vi "Vision_Right_R3.3.vi"() -> ()   [LabVIEW 2015]
uses:
  <vilib>/vision/Pattern Matching.llb/IMAQ Curve Parameters.ctl
  <vilib>/vision/Pattern Matching.llb/IMAQ Match Range Setting.ctl
  <vilib>/userdefined/High Color/IMAQdx.ctl
  <vilib>/vision/driver/NI_Vision_Acquisition_Software.lvlib
  <vilib>/vision/NI_Vision_Development_Module.lvlib
panel:
  in  "Range 0 Default\nSetting Values":T1={"Min Scale"=50.0, "Max Scale"=160.0, "Min Score"=850.0, "Lower Transition Scale"=45.0, "Upper Transition Scale"=200.0, "ROI Vertical"=2.0, "ROI Horizontal"=1.0, "Scale Cushion"=15.0, "Curve Parameters"={"Min Length"=15, "Row Search Step"=10, "Col Search Step"=10}, "Beacon Cushion (px)"=3.0, "Max Scale Diff\nfrom Main"=50.0}
  in  "Range 0 Templates":T2={"Sub - 2 File Path"=path "/home/lvuser/Beacon_Templates/Range_0/Range 0.png", "Sub Beacon Template File Path - ARRAY"=[path "/home/lvuser/Beacon_Templates/Range_1/Sub 0 - Range 1.png", path "/home/lvuser/Beacon_Templates/Range_1/Sub 1 - Range 1.png", path "/home/lvuser/Beacon_Templates/Range_1/Sub 2 - Range 1.png", path "/home/lvuser/Beacon_Templates/Range_1/Sub 3 - Range 1.png", path "/home/lvuser/Beacon_Templates/Range_1/Sub 4 - Range 1.png"]}
  in  "Correlation Score Threhsold (Range 0)":sgl=750.0
  in  "stop":bool
  in  "select (true= use advanced features\nfase= dont use)":bool
  in  "Range 3 Default\nSetting Values":T1={"Min Scale"=50.0, "Max Scale"=150.0, "Min Score"=800.0, "Lower Transition Scale"=1.0, "Upper Transition Scale"=130.0, "ROI Vertical"=3.5, "ROI Horizontal"=4.0, "Scale Cushion"=15.0, "Curve Parameters"={"Min Length"=2, "Row Search Step"=5, "Col Search Step"=5}, "Beacon Cushion (px)"=5.0, "Max Scale Diff\nfrom Main"=10.0}
  in  "Range 2 Default\nSetting Values":T1={"Min Scale"=65.0, "Max Scale"=130.0, "Min Score"=800.0, "Lower Transition Scale"=65.0, "Upper Transition Scale"=125.0, "ROI Vertical"=2.8, "ROI Horizontal"=4.0, "Scale Cushion"=17.0, "Curve Parameters"={"Min Length"=10, "Row Search Step"=10, "Col Search Step"=10}, "Beacon Cushion (px)"=15.0, "Max Scale Diff\nfrom Main"=20.0}
  in  "No Lock Default\nSetting Values":T3={"Min Scale"=25.0, "Max Scale"=200.0, "Min Score"=750.0, "Lower Transition Scale"=35.0, "Upper Transition Scale"=250.0, "ROI Vertical"=15.0, "ROI Horizontal"=15.0, "Scale Cushion"=15.0, "Curve Parameters"={"Min Length"=5, "Row Search Step"=10, "Col Search Step"=10}, "Scale Cushion 2"=15.0, "Max Scale Diff\nfrom Main"=15.0}
  in  "ROI Decay Factor (px)":dbl=50.0
  in  "ROBOT STATE\n(fwd, bwd, neither) 2":i32
  in  "Score Decay \nFactor 2":dbl=50.0
  in  "Range 1 Default\nSetting Values":T1={"Min Scale"=25.0, "Max Scale"=100.0, "Min Score"=800.0, "Lower Transition Scale"=35.0, "Upper Transition Scale"=67.0, "ROI Vertical"=0.75, "ROI Horizontal"=5.0, "Scale Cushion"=23.0, "Curve Parameters"={"Min Length"=15, "Row Search Step"=15, "Col Search Step"=15}, "Beacon Cushion (px)"=25.0, "Max Scale Diff\nfrom Main"=25.0}
  out "Next Template":T4(ring)
  out "Current Template":T4(ring)
  in  "Initial Template":T4(ring)
  in  "Range 3 Templates":T2={"Sub - 2 File Path"=path "/home/lvuser/Beacon_Templates/Range_3/5 Beacons - Range 3.png", "Sub Beacon Template File Path - ARRAY"=[path "/home/lvuser/Beacon_Templates/Range_3/Sub 0 - Range 3.png", path "/home/lvuser/Beacon_Templates/Range_3/Sub 1 - Range 3.png", path "/home/lvuser/Beacon_Templates/Range_3/Sub 2 - Range 3.png", path "/home/lvuser/Beacon_Templates/Range_3/Sub 3 - Range 3.png", path "/home/lvuser/Beacon_Templates/Range_3/Sub 4 - Range 3.png"]}
  in  "Range 2 Templates":T2={"Sub - 2 File Path"=path "/home/lvuser/Beacon_Templates/Range_2/5 Beacons - Range 2.png", "Sub Beacon Template File Path - ARRAY"=[path "/home/lvuser/Beacon_Templates/Range_2/Sub 0 - Range 2.png", path "/home/lvuser/Beacon_Templates/Range_2/Sub 1 - Range 2.png", path "/home/lvuser/Beacon_Templates/Range_2/Sub 2 - Range 2.png", path "/home/lvuser/Beacon_Templates/Range_2/Sub 3 - Range 2.png", path "/home/lvuser/Beacon_Templates/Range_2/Sub 4 - Range 2.png"]}
  in  "Range 1 Templates - RIGHT":T2={"Sub - 2 File Path"=path "/home/lvuser/Beacon_Templates/Range_1/2_Beacons_Right - Range 1.png", "Sub Beacon Template File Path - ARRAY"=[path "/home/lvuser/Beacon_Templates/Range_1/Sub 0 - Range 1.png", path "/home/lvuser/Beacon_Templates/Range_1/Sub 1 - Range 1.png", path "/home/lvuser/Beacon_Templates/Range_1/Sub 2 - Range 1.png", path "/home/lvuser/Beacon_Templates/Range_1/Sub 3 - Range 1.png", path "/home/lvuser/Beacon_Templates/Range_1/Sub 4 - Range 1.png"]}
  out "Current Correlation Score":sgl
  in  "Correlation Score Threhsold":sgl=300.0
  out "New Min Score":dbl=800.0
  out "New Low Scale":dbl=25.0
  out "New high Scale":dbl=100.0
  in  "Absolute\nMinimum Score":dbl=750.0
  in  "Absolute\nMaximum Scale":dbl=250.0
  in  "Absolute\nMinimum Scale":dbl=25.0
  in  "Score\nCushion":dbl=192.0
  in  "Avg Scale - Last":dbl=50.0
  in  "Avg Score - Last":dbl=986.6820373535156
  in  "Max Window\n for Avg":u8=3
  in  "Valid Treshold\nfor Lock":i16=3
  out "Current  Score":sgl
  out "Current  Scale":sgl
  out "Current Valid?":bool
  out "Beacon - Scales":sgl[](array[numeric])
  out "beacon - Scores":sgl[](array[numeric])
  out "Beacons Found":bool[](array[boolean])
  out "Horiztonall Beacon \nCushion (pixels)":sgl=25.0
  out "Tracking Info":T5={"Lock"=FALSE, "Current Valid"=FALSE, "Current Template"=enum."Range 1", "Tracking Coordinates"={"X"=159.0, "Y"=119.0}, "Setting Values"={"Min Score"=800.0, "Min Scale"=25.0, "Max Scale"=100.0, "Curve Parameters"={"Min Length"=15, "Row Search Step"=15, "Col Search Step"=15}}}
  out "dT":u32=629
  out "Avg Scale":dbl=50.0
  out "Avg Score":dbl=986.6820373535156
  out "Current Search Settings":T8={"Curve Parameters"={"Extraction Mode"=1, "Edge Threshold"=200, "Edge Filter Size"=0, "Min Length"=15, "Row Search Step Size"=15, "Col Search Step Size"=15, "Max Endpoint Gap"=4, "Closed"=TRUE, "Subpixel"=TRUE}, "Match Mode"={"Rotation"=TRUE, "Scale"=TRUE, "Occlusion"=TRUE, "Reserved"=FALSE, "Reserved"=FALSE, "Reserved"=FALSE}, "Range Settings"=[{"Match Constraints"=0, "Min"=-10.0, "Max"=2.0}, {"Match Constraints"=1, "Min"=25.0, "Max"=100.0}, {"Match Constraints"=2, "Min"=0.0, "Max"=20.0}], "Number of Matches"=1, "Minimum Match Score"=800.0, "SubPixel Accuracy"=TRUE, "Adv. Geometric Match Options 2"=[{"Setup Data Item"=20, "Item Value"=0.0}, {"Setup Data Item"=22, "Item Value"=1.0}]} {"Curve Parameters"."Extraction Mode" items=["Normal", "Uniform Regions"]; "Curve Parameters"."Edge Filter Size" items=["Fine", "Normal", "Contour Tracing"]; "Curve Parameters"."Max Endpoint Gap" min=0; "Curve Parameters"."Col Search Step Size" min=1 max=255 step=1; "Curve Parameters"."Row Search Step Size" min=1 max=255 step=1; "Curve Parameters"."Min Length" min=0; "Curve Parameters"."Edge Threshold" min=1 max=350 step=1; "Range Settings"."Max" format="%.2f"; "Range Settings"."Min" format="%.2f"; "Range Settings"."Match Constraints" items=["Rotation Angle (degrees)", "Scale Factor (%)", "Occlusion (%)"]}
  out "Valid Scale History":dbl[](array[numeric]) format="%#_13g"
  out "Valid Score History":dbl[](array[numeric]) format="%#_13g"
  out "Valid Beacon History - in":bool[](array[boolean])
  out "Startup Flag":bool
  out "Lock Status":bool
  out "Y Coordinates":sgl[](array[numeric])
  out "X Coordinates":sgl[](array[numeric])
  out "Right Image out":T9(plugin-control)
  in  "History Size":i32=19
  in  "INITIAL Search Settings":T8={"Curve Parameters"={"Extraction Mode"=1, "Edge Threshold"=200, "Edge Filter Size"=0, "Min Length"=15, "Row Search Step Size"=10, "Col Search Step Size"=10, "Max Endpoint Gap"=4, "Closed"=TRUE, "Subpixel"=TRUE}, "Match Mode"={"Rotation"=TRUE, "Scale"=TRUE, "Occlusion"=TRUE, "Reserved"=FALSE, "Reserved"=FALSE, "Reserved"=FALSE}, "Range Settings"=[{"Match Constraints"=0, "Min"=-10.0, "Max"=2.0}, {"Match Constraints"=1, "Min"=25.0, "Max"=150.0}, {"Match Constraints"=2, "Min"=0.0, "Max"=20.0}], "Number of Matches"=1, "Minimum Match Score"=750.0, "SubPixel Accuracy"=TRUE, "Adv. Geometric Match Options 2"=[{"Setup Data Item"=20, "Item Value"=0.0}, {"Setup Data Item"=22, "Item Value"=1.0}]} {"Curve Parameters"."Extraction Mode" items=["Normal", "Uniform Regions"]; "Curve Parameters"."Edge Filter Size" items=["Fine", "Normal", "Contour Tracing"]; "Curve Parameters"."Max Endpoint Gap" min=0; "Curve Parameters"."Col Search Step Size" min=1 max=255 step=1; "Curve Parameters"."Row Search Step Size" min=1 max=255 step=1; "Curve Parameters"."Min Length" min=0; "Curve Parameters"."Edge Threshold" min=1 max=350 step=1; "Range Settings"."Max" format="%.2f"; "Range Settings"."Min" format="%.2f"; "Range Settings"."Match Constraints" items=["Rotation Angle (degrees)", "Scale Factor (%)", "Occlusion (%)"]; "Adv. Geometric Match Options 2"."Setup Data Item" items=["Curve Extraction Mode", "Curve Edge Threshold", "Curve Edge Filter Size", "Min Curve Length", "Curve Row Search Step Size", "Curve Col Search Step Size", "Curve Max Endpoint Gap", "Extract Closed Curves", "Enable Subpixel Curve Extraction", "Enable Correlation Score", "Enable Subpixel Accuracy", "Subpixel Iterations", "Subpixel Tolerance", "Initial Match List Length", "Enable Target Template Curve Score", "Min Match Separation Distance", "Min Match Separation Angle", "Min Match Separation Scale", "Max Match Overlap", "Enable Coarse Result", "Enable Calibration Support", "Enable Contrast Reversal", "Search Strategy", "Refinement Match Factor", "Subpixel Match Factor"]}
  # "ROI Factore (per Template)"
  # "Template Transition Scales"
  # "Search Parameter Limits"
  # "TEMPLATE FILE PATHS"
  # "Config"
  # "Initial Settings"
  # "Range"
  # "Range"
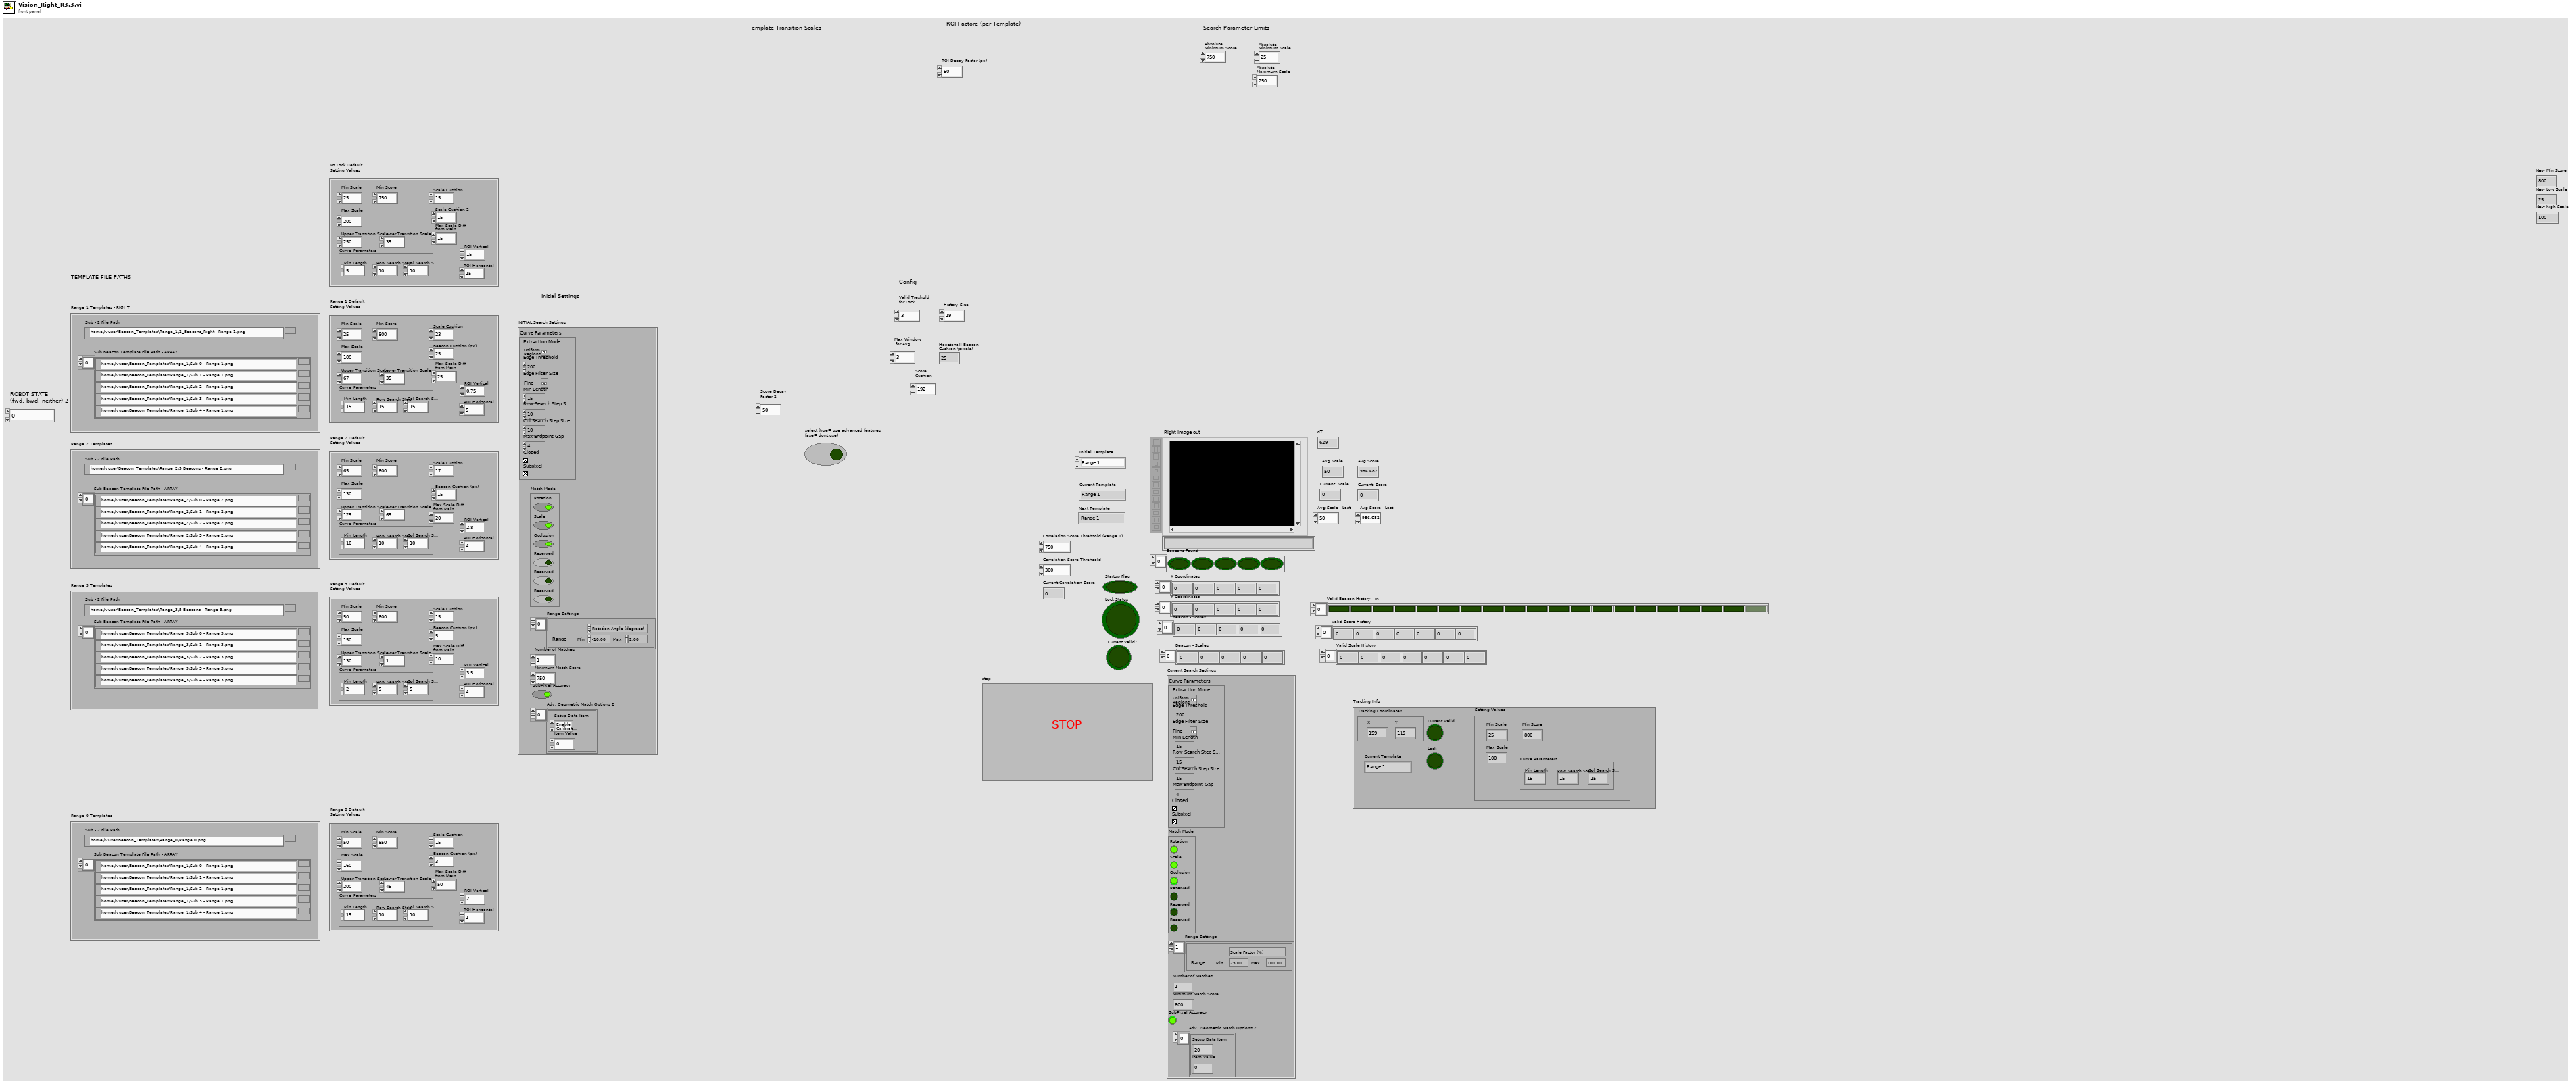
[diagram p1: front panel]
types:
  T1 = cluster{"Min Scale":dbl, "Max Scale":dbl, "Min Score":dbl, "Lower Transition Scale":sgl, "Upper Transition Scale":sgl, "ROI Vertical":dbl, "ROI Horizontal":dbl, "Scale Cushion":dbl, "Curve Parameters":cluster{"Min Length":i32, "Row Search Step":i32, "Col Search Step":i32}, "Beacon Cushion (px)":dbl, "Max Scale Diff\nfrom Main":dbl}
  T2 = cluster{"Sub - 2 File Path":path, "Sub Beacon Template File Path - ARRAY":path[]}
  T3 = cluster{"Min Scale":dbl, "Max Scale":dbl, "Min Score":dbl, "Lower Transition Scale":sgl, "Upper Transition Scale":sgl, "ROI Vertical":dbl, "ROI Horizontal":dbl, "Scale Cushion":dbl, "Curve Parameters":cluster{"Min Length":i32, "Row Search Step":i32, "Col Search Step":i32}, "Scale Cushion 2":dbl, "Max Scale Diff\nfrom Main":dbl}
  T4 = enum16{"Range 1", "Range 2", "Range 3", "Range 0"}
  T5 = cluster{"Lock":bool, "Current Valid":bool, "Current Template":enum16{"Range 1", "Range 2", "Range 3", "Range 0"}, "Tracking Coordinates":cluster{"X":dbl, "Y":dbl}, "Setting Values":cluster{"Min Score":dbl, "Min Scale":dbl, "Max Scale":dbl, "Curve Parameters":cluster{"Min Length":i32, "Row Search Step":i32, "Col Search Step":i32}}}
  T6 = typedef "IMAQ Curve Parameters.ctl" = cluster{"Extraction Mode":u32, "Edge Threshold":i32, "Edge Filter Size":u32, "Min Length":i32, "Row Search Step Size":i32, "Col Search Step Size":i32, "Max Endpoint Gap":i32, "Closed":bool, "Subpixel":bool}
  T7 = typedef "IMAQ Match Range Setting.ctl" = cluster{"Match Constraints":u32, "Min":dbl, "Max":dbl}
  T8 = cluster{"Curve Parameters":T6, "Match Mode":cluster{"Rotation":bool, "Scale":bool, "Occlusion":bool, "Reserved":bool, "Reserved":bool, "Reserved":bool}, "Range Settings":T7[], "Number of Matches":i32, "Minimum Match Score":sgl, "SubPixel Accuracy":bool, "Adv. Geometric Match Options 2":cluster{"Setup Data Item":u16, "Item Value":dbl}[]}
  T9 = typedef "IMAQ Image.ctl" = refnum<image>
  T10 = typedef "IMAQdx.ctl" = refnum<k21>
  T11 = typedef "Image Type" = u32
  T12 = typedef "ROI Descriptor" = cluster{"Global Rectangle":i32[], "Contours":cluster{"ID":enum32{"External", "Internal"}, "Type":u32, "Coordinates":i32[]}[]}
  T13 = typedef "IMAQ GM Match Report.ctl" = cluster{"Position":cluster{"x":sgl, "y":sgl}, "Angle":sgl, "Scale":sgl, "Score":sgl, "Bounding Box":cluster{"x":sgl, "y":sgl}[], "Contrast Reversed":bool, "Occlusion %":sgl, "Template Target Curve Score":sgl, "Target Template Curve Score":sgl, "Correlation Score":sgl}
  T14 = cluster{"Matches[0]":T13, "Matches[1]":T13, "Matches[2]":T13, "Matches[3]":T13, "Matches[4]":T13, "Matches[5]":T13, "Matches[6]":T13, "Matches[7]":T13, "Matches[8]":T13}
  T15 = cluster{"Bounding Box[0]":cluster{"x":sgl, "y":sgl}, "Bounding Box[1]":cluster{"x":sgl, "y":sgl}, "Bounding Box[2]":cluster{"x":sgl, "y":sgl}, "Bounding Box[3]":cluster{"x":sgl, "y":sgl}, "Bounding Box[4]":cluster{"x":sgl, "y":sgl}, "Bounding Box[5]":cluster{"x":sgl, "y":sgl}, "Bounding Box[6]":cluster{"x":sgl, "y":sgl}, "Bounding Box[7]":cluster{"x":sgl, "y":sgl}, "Bounding Box[8]":cluster{"x":sgl, "y":sgl}}
  T16 = cluster{"Matches (Geometric Matching 1)[0]":T13, "Matches (Geometric Matching 1)[1]":T13, "Matches (Geometric Matching 1)[2]":T13, "Matches (Geometric Matching 1)[3]":T13, "Matches (Geometric Matching 1)[4]":T13, "Matches (Geometric Matching 1)[5]":T13, "Matches (Geometric Matching 1)[6]":T13, "Matches (Geometric Matching 1)[7]":T13, "Matches (Geometric Matching 1)[8]":T13}
  T17 = cluster{"Min Length":i32, "Row Search Step":i32, "Col Search Step":i32}
  T18 = cluster{"Extraction Mode":u32, "Edge Threshold":i32, "Edge Filter Size":u32, "Min Length":i32, "Row Search Step":i32, "Col Search Step":i32, "Max Endpoint Gap":i32, "Closed":bool, "Subpixel":bool}
  T19 = typedef "IMAQ Rectangle" = cluster{"Left":i32, "Top":i32, "Right":i32, "Bottom":i32, "Rotation":dbl}
  T20 = cluster{"Min Length":i32, "Row Search Step Size":i32, "Col Search Step Size":i32}
  T21 = cluster{"Min Score":dbl, "Min":dbl, "Max":dbl, cluster{"Min Length":i32, "Row Search Step Size":i32, "Col Search Step Size":i32}}
  T22 = cluster{bool, bool, "Initial Template":enum16{"Range 1", "Range 2", "Range 3", "Range 0"}, "Position":cluster{"x":dbl, "y":dbl}, cluster{"Min Score":dbl, "Min":dbl, "Max":dbl, cluster{"Min Length":i32, "Row Search Step Size":i32, "Col Search Step Size":i32}}}
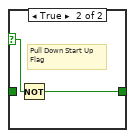
[diagram p2: hidden frame]
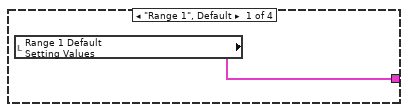
[diagram p3: hidden frame]
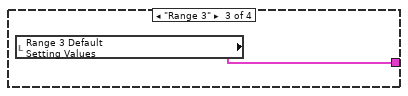
[diagram p4: hidden frame]
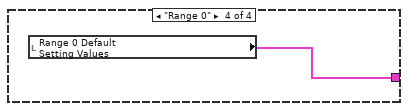
[diagram p5: hidden frame]
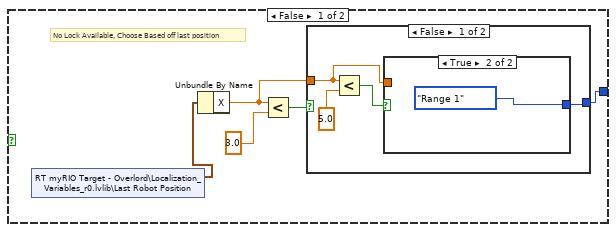
[diagram p6: hidden frame]
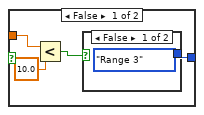
[diagram p7: hidden frame]
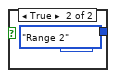
[diagram p8: hidden frame]
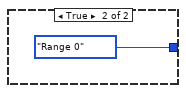
[diagram p9: hidden frame]
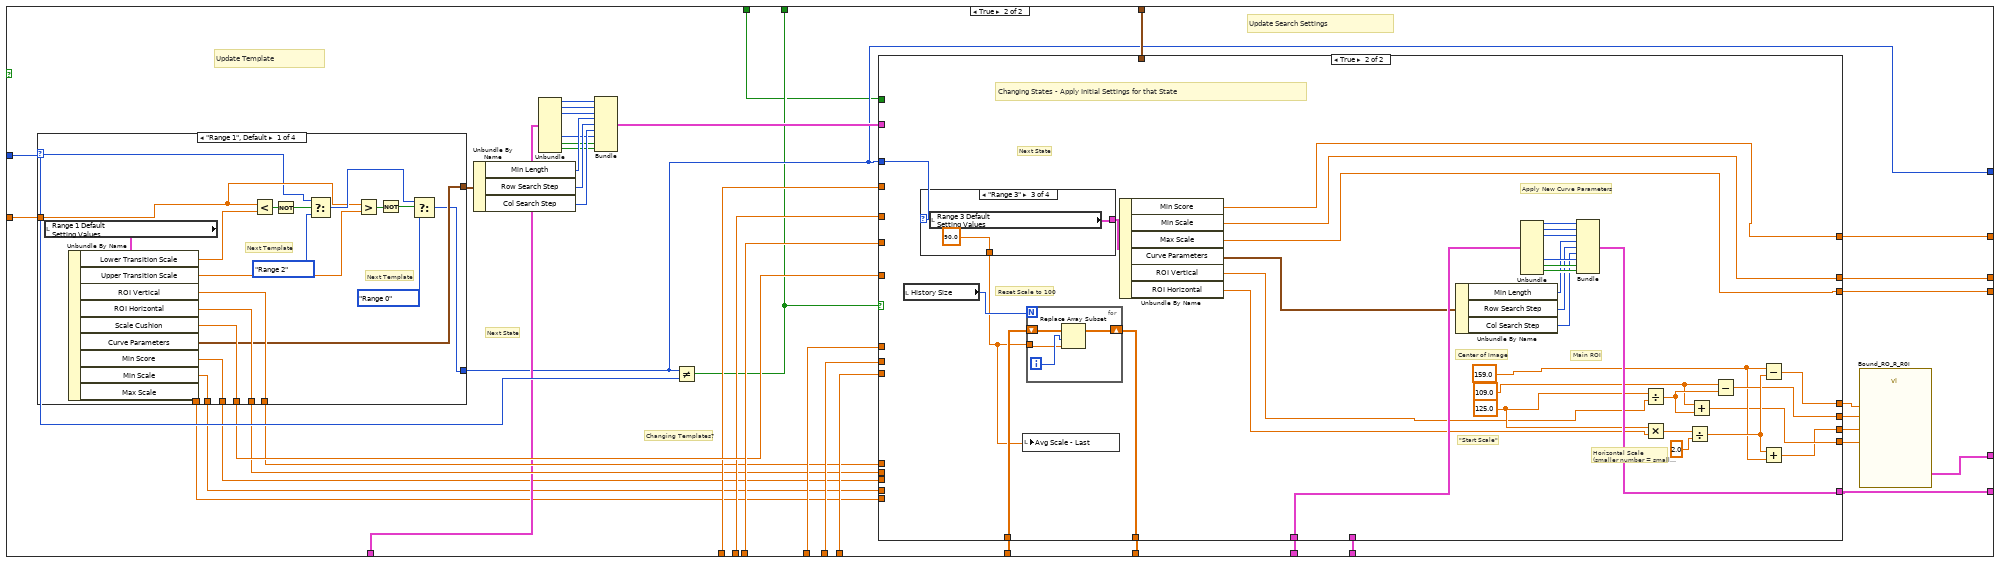
[diagram p10: hidden frame]
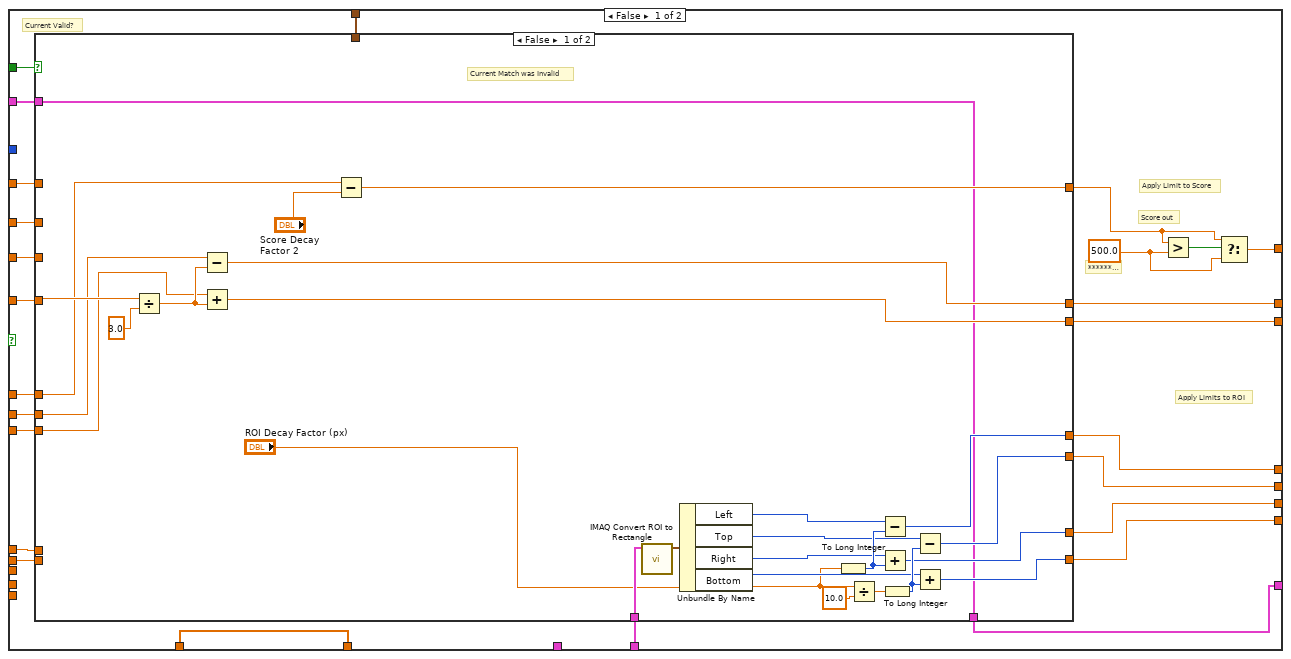
[diagram p11: hidden frame]
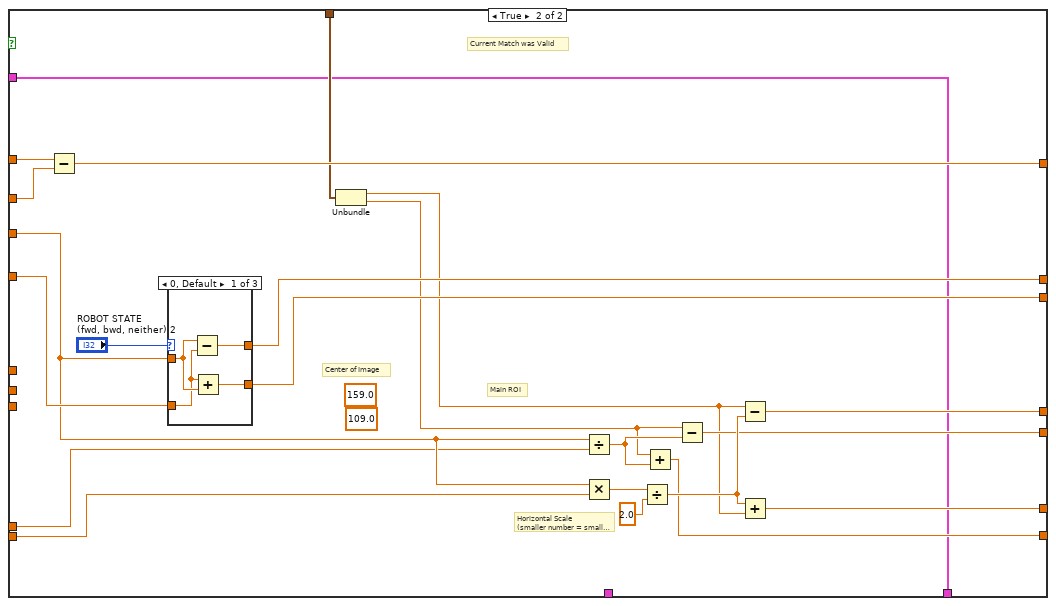
[diagram p12: hidden frame]
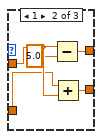
[diagram p13: hidden frame]
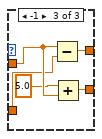
[diagram p14: hidden frame]
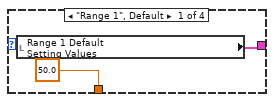
[diagram p15: hidden frame]
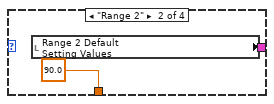
[diagram p16: hidden frame]
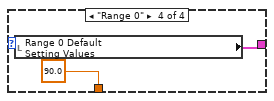
[diagram p17: hidden frame]
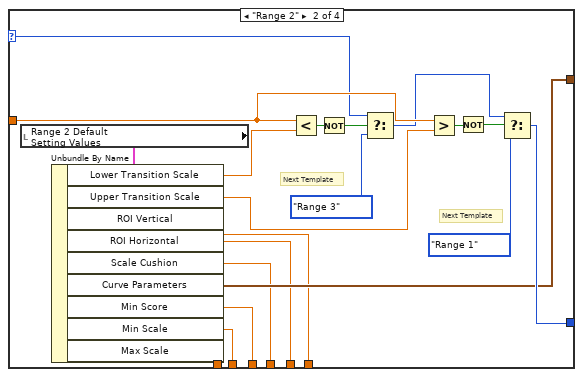
[diagram p18: hidden frame]
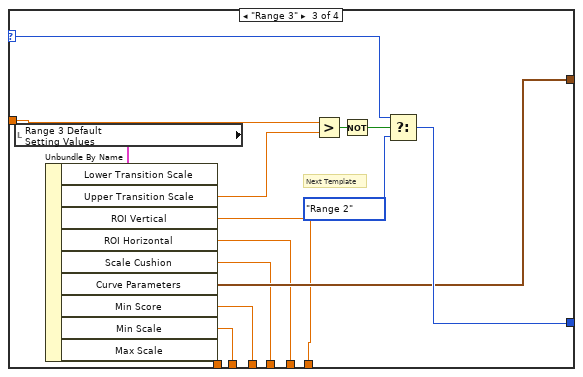
[diagram p19: hidden frame]
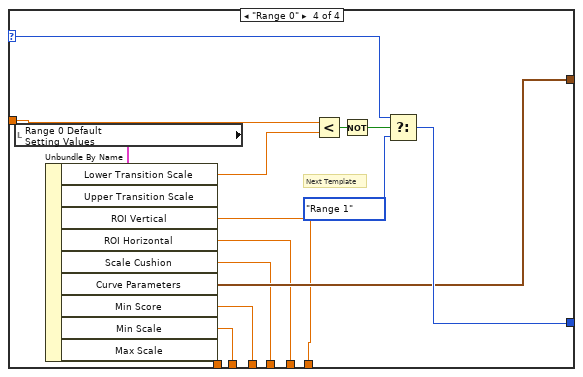
[diagram p20: hidden frame]
diagram:
  n1 = flat-sequence {
    tunnel: [w38] -> w16
    tunnel: ["INITIAL Search Settings"] -> w15
    tunnel: ["Initial Template"] -> w14
    tunnel: [TRUE] -> w13
    tunnel: [w35] -> w12
    tunnel: [w34] -> w11
    tunnel: [w33] -> w10
    tunnel: [w32] -> w9
    tunnel: [w31] -> w8
    tunnel: ["History Size"] -> w7
    tunnel: [750.0] -> w6
    tunnel: [100.0] -> w5
    tunnel: [w19] -> w4
    tunnel: [w18] -> w3
    tunnel: [w17] -> w2
    tunnel: w16 -> [w64]
    tunnel: w15 -> [w63]
    tunnel: w14 -> [w62]
    tunnel: w13 -> [w61]
    tunnel: w12 -> [w57]
    tunnel: w11 -> [w54]
    tunnel: w10 -> [w60]
    tunnel: w9 -> [w59]
    tunnel: w8 -> [w58]
    tunnel: w7 -> [w56]
    tunnel: w6 -> [_]
    tunnel: w5 -> [_]
    tunnel: w4 -> [w53]
    tunnel: w3 -> [w52]
    tunnel: w2 -> [w51]
    tunnel: [w50] -> w1
    tunnel: w1 -> [w863]
    frame #0 {
      w24 = "[NIIMAQ_HEADER]\nType = 2\nVersion = 8\n\n[CAMERA_DATA]\nAcquisitionAttributes::Bayer::Algorithm = \"Bilinear\"\nAcquisitionAttributes::Bayer::GainB = \"1\"\nAcquisitionAttributes::Bayer::GainG = \"1\"\nAcquisitionAttributes::Bayer::GainR = \"1\"\nAcquisitionAttributes::Bayer::Pattern = \"Use hardware value\"\nAcquisitionAttributes::BitsPerPixel = \"Use hardware value\"\nAcquisitionAttributes::IgnoreFirstFrame = \"false\"\nAcquisitionAttributes::ImageDecoderCopyMode = \"Auto\"\nAcquisitionAttributes::OutputImageType = \"Auto\"\nAcquisitionAttributes::OverwriteMode = \"Get Newest\"\nAcquisitionAttributes::PixelSignedness = \"Use hardware value\"\nAcquisitionAttributes::ReceiveTimestampMode = \"None\"\nAcquisitionAttributes::ShiftPixelBits = \"false\"\nAcquisitionAttributes::SwapPixelBytes = \"false\"\nAcquisitionAttributes::Timeout = \"5000\"\nAcquisitionAttributes::VerticalMirror = \"false\"\nAcquisitionAttributes::VideoMode = \"320x240 YUY2 30.00fps\"\nCameraAttributes::BacklightCompensation::Mode = \"Manual\"\nCameraAttributes::BacklightCompensation::Value = \"false\"\nCameraAttributes::Brightness::Mode = \"UnknownEnumValue\"\nCameraAttributes::Brightness::Value = \"133\"\nCameraAttributes::Contrast::Mode = \"Manual\"\nCameraAttributes::Contrast::Value = \"0\"\nCameraAttributes::Exposure::Mode = \"Auto\"\nCameraAttributes::Focus::Mode = \"Auto\"\nCameraAttributes::Pan::Mode = \"Manual\"\nCameraAttributes::Pan::Value = \"0\"\nCameraAttributes::Saturation::Mode = \"Manual\"\nCameraAttributes::Saturation::Value = \"103\"\nCameraAttributes::Sharpness::Mode = \"Manual\"\nCameraAttributes::Sharpness::Value = \"25\"\nCameraAttributes::Tilt::Mode = \"Manual\"\nCameraAttributes::Tilt::Value = \"0\"\nCameraAttributes::WhiteBalance::Mode = \"Auto\"\nCameraAttributes::Zoom::Mode = \"Manual\"\nCameraAttributes::Zoom::Value = \"0\"\n"  # Attributes
      w45 = T11 0 items=["Grayscale (U8)", "Grayscale (I16)", "Grayscale (SGL)", "Complex (CSG)", "RGB (U32)", "HSL (U32)", "RGB (U64)", "Grayscale (U16)"] ("Image Type")
      # "avg start scale"
      # "Score History"
      # "Scale History"
      # "Valid Match History\n(main beacon)"
      # "Template State"
      # "Search Parameters"
      # "StartUp = True"
      # "Initial ROI Descriptor"
      # "INITIALIZE"
      n2 = call <vilib>:"IMAQdx Open Camera.vi"("Session In"=T10 "cam0") -> ("error out"=w22:errorcluster, "Session Out"=w23:T10)  [unwired: 2 in, 7 out]
      n3 = call <vilib>:"IMAQdx Read Attributes From String.vi"("error in"=w22, "Attributes String In"=w24, "Session In"=w23) -> ("error out"=w21:errorcluster, "Session Out"=w20:T10)  [unwired: 7 out]
      n4 = Bundle(0, 0, 640, 480, 0) -> (w44:cluster{i32, i32, i32, i32, i32})  [unwired: 1 in]
      n5 = call "IMAQ Convert Rectangle to ROI"("Rectangle"=w44) -> ("ROI Descriptor"=w38:T12)  [unwired: 8 in, 1 out]
      n6 = call "IMAQ Create"("Image Name"="Right_Image", "Image Type"=w45) -> ("New Image"=w35:T9, "error out"=w34:errorcluster)  [unwired: 3 in]
      n7 = Initialize Array(FALSE, "History Size") -> (w33:bool[])
      n8 = Initialize Array(0.0, "History Size") -> (w31:dbl[])
      n9 = Initialize Array(0.0, "History Size") -> (w32:dbl[])
      n10 = call <vilib>:"IMAQdx Configure Grab.vi"("error in"=w21, "Session In"=w20) -> ("error out"=w17:errorcluster, "Session Out"=w19:T10)  [unwired: 8 in]
      n11 = call "IMAQ Create"("Image Name"="Original") -> ("New Image"=w18:T9)  [unwired: 4 in, 1 out]
    }
    frame #1 {
      # "Avg Scale"
      # "Avg Score"
      # "Score History"
      # "Scale History"
      # "Valid Match History\n(main beacon)"
      # "Sub Beacon Search Array"
      # "StartUp = True"
      # "Template State"
      # "Search Parameters"
      # "ROI"
      n12 = call "Tick Count"() -> ("Tick Count(mSec)"=w55:u32)
      n13 = while {
        shift-right: [w77] -> _
        shift-left: w64 -> [w91]
        shift-right: [w87] -> _
        shift-left: w63 -> [w92]
        shift-right: [w76] -> _
        shift-left: w62 -> [w79]
        shift-right: [w74] -> _
        shift-left: w61 -> [w75]
        shift-right: [w83] -> _
        shift-left: w60 -> [w84]
        shift-right: [w73] -> _
        shift-left: w59 -> [w82]
        shift-right: [w80] -> _
        shift-left: w58 -> [w81]
        shift-right: [w86] -> _
        shift-left: w57 -> [w93]
        tunnel: w56 -> [w98]
        shift-right: [w96] -> _
        shift-left: w55 -> [w97]
        tunnel: w54 -> [w85]
        tunnel: w53 -> [w72]
        tunnel: w52 -> [w71]
        tunnel: w51 -> [w70]
        tunnel: [w67] -> w50
        stop <- "stop" stop-if-true
        n14 = call "Tick Count2"() -> ("Tick Count(mSec)"=w96:u32)
        n15 = Subtract(x=w96, y=w97) -> (x-y=→"dT":u32)
        n16 = flat-sequence {
          tunnel: [w99] -> w89
          tunnel: [w106] -> w94
          tunnel: w93 -> [w106]
          tunnel: [w106] -> w86
          tunnel: w85 -> [_]
          tunnel: w72 -> [w105]
          tunnel: w71 -> [w104]
          tunnel: w70 -> [w103]
          tunnel: [w102] -> w69
          tunnel: [w101] -> w68
          tunnel: [w100] -> w66
          tunnel: w79 -> [w117]
          tunnel: w84 -> [w224]
          tunnel: w82 -> [w223]
          tunnel: w81 -> [w222]
          tunnel: w98 -> [_]
          tunnel: w94 -> [w128]
          tunnel: w92 -> [w129]
          tunnel: w91 -> [w131]
          tunnel: [w191] -> w90
          tunnel: w89 -> [w184]
          tunnel: [w184] -> w88
          tunnel: [w183] -> w83
          tunnel: [w151] -> _
          tunnel: [w182] -> w80
          tunnel: w75 -> [w149]
          tunnel: [w153] -> w78
          tunnel: [w154] -> w77
          tunnel: [w153] -> w76
          tunnel: [w148] -> w74
          tunnel: [w152] -> w73
          tunnel: w69 -> [w123]
          tunnel: w68 -> [w122]
          tunnel: [w121] -> w67
          tunnel: w66 -> [w121]
          tunnel: w90 -> [w862]
          tunnel: w88 -> [w860]
          tunnel: [w862] -> w87
          tunnel: [w861] -> _
          tunnel: w78 -> [w861]
          frame #0 {
            # "Aquire Image"
            n17 = shared-variable "RT myRIO Target - Overlord\\Localization_Variables_r0.lvlib\\Right Servo Angle_Current"() -> (w99:dbl)  [unwired: 1 in, 1 out]
            n18 = call <vilib>:"IMAQdx Grab2.vi"("error in"=w103, "Image In"=w104, "Session In"=w105) -> ("error out"=w101:errorcluster, "Image Out"=w102:T9, "Session Out"=w100:T10)  [unwired: 5 in, 1 out]
          }
          frame #1 {
            (unwired) T4."Range 1" ("Initial Template 2")
            w141 = 6 items=["Red", "Green", "Blue", "Hue", "Saturation", "Luminance", "Value", "Intensity"] ("Color Plane")
            w194 = u32 1 ("index")
            # "Tracking Position"
            # "ROI center"
            # "Add mode when CLose to look for all individual beacons with full ROI"
            # "Service Start Up Flag"
            # "Change States?"
            # "Next Template"
            # "Max Scale"
            # "Min Scale"
            # "Min Score"
            # "Curve p"
            # "ROI"
            # "Current Scale Range"
            # "Current Min Score"
            # "Avg Score"
            # "Avg Scale"
            # "Startup?"
            # "********** Look into False case **********"
            # "SUm # of Sub-Beacons Found, Check if Enoough\nto be considered Valid"
            # "Update Tracking Coordinates"
            # "Next Settings"
            # "Current Settings"
            # "Current Min\n& Max Scale"
            # "Scale"
            # "Min Score"
            # "Lower Scale"
            # "Upper Scale"
            # "Min Score out"
            # "Score History"
            # "Min Required to use avarage"
            # "Scale History"
            # "History Size"
            # "Calculate Average Score/Scale"
            # "****# of previous in history that must be true\nin order for position to be considered \"locked\""
            # "Scale History"
            # "Score History"
            # "Valid History"
            # "Update History Data"
            # "1 Match FOund?"
            # "# of Sub Beacons"
            # "Sub Beacons to Search For"
            # "# Sub Beacons to Find in\norder to be valid"
            # "Template Filepath & Sub Beacon Array"
            # "Select Current Template Config"
            # "Pattern Match to Current Template"
            # "Apply FIltering"
            n19 = call "IMAQ ImageBorderSize"("Get/Set Status? (Set)"=TRUE, "Image"=w123, "Image border size in"=13 ("Border Size"), "error in (no error)"=w122) -> ("Image Out"=w140:T9, "error out"=w144:errorcluster)  [unwired: 1 out]
            n20 = call "IMAQ ExtractSingleColorPlane"("Color Plane"=w141, "error in (no error)"=w144, "Image Src"=w140) -> ("error out"=w139:errorcluster, "Image Dst Out"=w137:T9)  [unwired: 1 in, 6 out]
            n21 = call "IMAQ Convolute"("Kernel"=sgl[][] [[1.0, 2.0, 1.0], [2.0, 4.0, 2.0], [1.0, 2.0, 1.0]], "Divider (kernel sum)"=sgl 9.0 ("Divider"), "error in (no error)"=w139, "Image Src"=w137) -> ("error out"=w136:errorcluster, "Image Dst Out"=w133:T9)  [unwired: 3 in, 3 out]
            n22 = call "IMAQ Convolute"("Kernel"=sgl[][] [[-1.0, -1.0, -1.0, -1.0, -1.0, -1.0, -1.0, -1.0, -1.0, -1.0, -1.0, -1.0, -1.0, -1.0, -1.0, -1.0, -1.0, -1.0, -1.0, -1.0, -1.0, -1.0, -1.0, -1.0, -1.0, -1.0, -1.0], [-1.0, -1.0, -1.0, -1.0, -1.0, -1.0, -1.0, -1.0, -1.0, -1.0, -1.0, -1.0, -1.0, -1.0, -1.0, -1.0, -1.0, -1.0, -1.0, -1.0, -1.0, -1.0, -1.0, -1.0, -1.0, -1.0, -1.0], [-1.0, -1.0, -1.0, -1.0, -1.0, -1.0, -1.0, -1.0, -1.0, -1.0, -1.0, -1.0, -1.0, -1.0, -1.0, -1.0, -1.0, -1.0, -1.0, -1.0, -1.0, -1.0, -1.0, -1.0, -1.0, -1.0, -1.0], [-1.0, -1.0, -1.0, -1.0, -1.0, -1.0, -1.0, -1.0, -1.0, -1.0, -1.0, -1.0, -1.0, -1.0, -1.0, -1.0, -1.0, -1.0, -1.0, -1.0, -1.0, -1.0, -1.0, -1.0, -1.0, -1.0, -1.0], [-1.0, -1.0, -1.0, -1.0, -1.0, -1.0, -1.0, -1.0, -1.0, -1.0, -1.0, -1.0, -1.0, -1.0, -1.0, -1.0, -1.0, -1.0, -1.0, -1.0, -1.0, -1.0, -1.0, -1.0, -1.0, -1.0, -1.0], [-1.0, -1.0, -1.0, -1.0, -1.0, -1.0, -1.0, -1.0, -1.0, -1.0, -1.0, -1.0, -1.0, -1.0, -1.0, -1.0, -1.0, -1.0, -1.0, -1.0, -1.0, -1.0, -1.0, -1.0, -1.0, -1.0, -1.0], [-1.0, -1.0, -1.0, -1.0, -1.0, -1.0, -1.0, -1.0, -1.0, -1.0, -1.0, -1.0, -1.0, -1.0, -1.0, -1.0, -1.0, -1.0, -1.0, -1.0, -1.0, -1.0, -1.0, -1.0, -1.0, -1.0, -1.0], [-1.0, -1.0, -1.0, -1.0, -1.0, -1.0, -1.0, -1.0, -1.0, -1.0, -1.0, -1.0, -1.0, -1.0, -1.0, -1.0, -1.0, -1.0, -1.0, -1.0, -1.0, -1.0, -1.0, -1.0, -1.0, -1.0, -1.0], [-1.0, -1.0, -1.0, -1.0, -1.0, -1.0, -1.0, -1.0, -1.0, -1.0, -1.0, -1.0, -1.0, -1.0, -1.0, -1.0, -1.0, -1.0, -1.0, -1.0, -1.0, -1.0, -1.0, -1.0, -1.0, -1.0, -1.0], [-1.0, -1.0, -1.0, -1.0, -1.0, -1.0, -1.0, -1.0, -1.0, -1.0, -1.0, -1.0, -1.0, -1.0, -1.0, -1.0, -1.0, -1.0, -1.0, -1.0, -1.0, -1.0, -1.0, -1.0, -1.0, -1.0, -1.0], [-1.0, -1.0, -1.0, -1.0, -1.0, -1.0, -1.0, -1.0, -1.0, -1.0, -1.0, -1.0, -1.0, -1.0, -1.0, -1.0, -1.0, -1.0, -1.0, -1.0, -1.0, -1.0, -1.0, -1.0, -1.0, -1.0, -1.0], [-1.0, -1.0, -1.0, -1.0, -1.0, -1.0, -1.0, -1.0, -1.0, -1.0, -1.0, -1.0, -1.0, -1.0, -1.0, -1.0, -1.0, -1.0, -1.0, -1.0, -1.0, -1.0, -1.0, -1.0, -1.0, -1.0, -1.0], [-1.0, -1.0, -1.0, -1.0, -1.0, -1.0, -1.0, -1.0, -1.0, -1.0, -1.0, -1.0, -1.0, -1.0, -1.0, -1.0, -1.0, -1.0, -1.0, -1.0, -1.0, -1.0, -1.0, -1.0, -1.0, -1.0, -1.0], [-1.0, -1.0, -1.0, -1.0, -1.0, -1.0, -1.0, -1.0, -1.0, -1.0, -1.0, -1.0, -1.0, 728.0, -1.0, -1.0, -1.0, -1.0, -1.0, -1.0, -1.0, -1.0, -1.0, -1.0, -1.0, -1.0, -1.0], [-1.0, -1.0, -1.0, -1.0, -1.0, -1.0, -1.0, -1.0, -1.0, -1.0, -1.0, -1.0, -1.0, -1.0, -1.0, -1.0, -1.0, -1.0, -1.0, -1.0, -1.0, -1.0, -1.0, -1.0, -1.0, -1.0, -1.0], [-1.0, -1.0, -1.0, -1.0, -1.0, -1.0, -1.0, -1.0, -1.0, -1.0, -1.0, -1.0, -1.0, -1.0, -1.0, -1.0, -1.0, -1.0, -1.0, -1.0, -1.0, -1.0, -1.0, -1.0, -1.0, -1.0, -1.0], [-1.0, -1.0, -1.0, -1.0, -1.0, -1.0, -1.0, -1.0, -1.0, -1.0, -1.0, -1.0, -1.0, -1.0, -1.0, -1.0, -1.0, -1.0, -1.0, -1.0, -1.0, -1.0, -1.0, -1.0, -1.0, -1.0, -1.0], [-1.0, -1.0, -1.0, -1.0, -1.0, -1.0, -1.0, -1.0, -1.0, -1.0, -1.0, -1.0, -1.0, -1.0, -1.0, -1.0, -1.0, -1.0, -1.0, -1.0, -1.0, -1.0, -1.0, -1.0, -1.0, -1.0, -1.0], [-1.0, -1.0, -1.0, -1.0, -1.0, -1.0, -1.0, -1.0, -1.0, -1.0, -1.0, -1.0, -1.0, -1.0, -1.0, -1.0, -1.0, -1.0, -1.0, -1.0, -1.0, -1.0, -1.0, -1.0, -1.0, -1.0, -1.0], [-1.0, -1.0, -1.0, -1.0, -1.0, -1.0, -1.0, -1.0, -1.0, -1.0, -1.0, -1.0, -1.0, -1.0, -1.0, -1.0, -1.0, -1.0, -1.0, -1.0, -1.0, -1.0, -1.0, -1.0, -1.0, -1.0, -1.0], [-1.0, -1.0, -1.0, -1.0, -1.0, -1.0, -1.0, -1.0, -1.0, -1.0, -1.0, -1.0, -1.0, -1.0, -1.0, -1.0, -1.0, -1.0, -1.0, -1.0, -1.0, -1.0, -1.0, -1.0, -1.0, -1.0, -1.0], [-1.0, -1.0, -1.0, -1.0, -1.0, -1.0, -1.0, -1.0, -1.0, -1.0, -1.0, -1.0, -1.0, -1.0, -1.0, -1.0, -1.0, -1.0, -1.0, -1.0, -1.0, -1.0, -1.0, -1.0, -1.0, -1.0, -1.0], [-1.0, -1.0, -1.0, -1.0, -1.0, -1.0, -1.0, -1.0, -1.0, -1.0, -1.0, -1.0, -1.0, -1.0, -1.0, -1.0, -1.0, -1.0, -1.0, -1.0, -1.0, -1.0, -1.0, -1.0, -1.0, -1.0, -1.0], [-1.0, -1.0, -1.0, -1.0, -1.0, -1.0, -1.0, -1.0, -1.0, -1.0, -1.0, -1.0, -1.0, -1.0, -1.0, -1.0, -1.0, -1.0, -1.0, -1.0, -1.0, -1.0, -1.0, -1.0, -1.0, -1.0, -1.0], [-1.0, -1.0, -1.0, -1.0, -1.0, -1.0, -1.0, -1.0, -1.0, -1.0, -1.0, -1.0, -1.0, -1.0, -1.0, -1.0, -1.0, -1.0, -1.0, -1.0, -1.0, -1.0, -1.0, -1.0, -1.0, -1.0, -1.0], [-1.0, -1.0, -1.0, -1.0, -1.0, -1.0, -1.0, -1.0, -1.0, -1.0, -1.0, -1.0, -1.0, -1.0, -1.0, -1.0, -1.0, -1.0, -1.0, -1.0, -1.0, -1.0, -1.0, -1.0, -1.0, -1.0, -1.0], [-1.0, -1.0, -1.0, -1.0, -1.0, -1.0, -1.0, -1.0, -1.0, -1.0, -1.0, -1.0, -1.0, -1.0, -1.0, -1.0, -1.0, -1.0, -1.0, -1.0, -1.0, -1.0, -1.0, -1.0, -1.0, -1.0, -1.0]], "Divider (kernel sum)"=sgl 10.0 ("Divider"), "error in (no error)"=w136, "Image Src"=w133) -> ("error out"=w146:errorcluster, "Image Dst Out"=w145:T9)  [unwired: 3 in, 3 out]
            n23 = case shown="\"Range 1\", Default" w117 {
              tunnel: ["Range 1 Templates - RIGHT" "Range 0 Templates" "Range 2 Templates" "Range 3 Templates"] -> w176
              tunnel: [w567 w574 w586 w593] -> w174
              tunnel: [sgl 2.0 sgl 0.0 sgl 5.0 sgl 5.0] -> w173
              tunnel: [1 1 3 3] -> w172
              tunnel: [w564 w578 w582 w591] -> w119
              tunnel: "Correlation Score Threhsold" -> [w564 _ w582 w591]
              tunnel: "Correlation Score Threhsold (Range 0)" -> [_ w578 _ _]
              tunnel: [w562 w572 w580 w589] -> w114
              tunnel: [w561 w570 w579 w588] -> w113
              frame "Range 1", Default {
                w568 = TRUE
                w560 = FALSE
                n24 = Unbundle By Name("Range 1 Default\nSetting Values") -> ("Max Scale Diff\nfrom Main"=w562:dbl, "Beacon Cushion (px)"=w561:dbl)
                n25 = Build Array(w560, w560, w560, w568, w568) -> (w567:bool[])
              }
              frame "Range 0" {
                (unwired) TRUE
                w575 = FALSE
                n26 = Unbundle By Name("Range 0 Default\nSetting Values") -> ("Max Scale Diff\nfrom Main"=w572:dbl, "Beacon Cushion (px)"=w570:dbl)
                n27 = Build Array(w575, w575, w575, w575, w575) -> (w574:bool[])
              }
              frame "Range 2" {
                (unwired) FALSE
                w587 = TRUE
                n28 = Unbundle By Name("Range 2 Default\nSetting Values") -> ("Max Scale Diff\nfrom Main"=w580:dbl, "Beacon Cushion (px)"=w579:dbl)
                n29 = Build Array(w587, w587, w587, w587, w587) -> (w586:bool[])
              }
              frame "Range 3" {
                (unwired) FALSE
                w594 = TRUE
                n30 = Unbundle By Name("Range 3 Default\nSetting Values") -> ("Max Scale Diff\nfrom Main"=w589:dbl, "Beacon Cushion (px)"=w588:dbl)
                n31 = Build Array(w594, w594, w594, w594, w594) -> (w593:bool[])
              }
            }
            n32 = Unbundle(w176) -> ("Sub - 2 File Path"=w130:path, "Sub Beacon Template File Path - ARRAY"=w175:path[])
            n33 = call "pattern_match_subvi.vi"("Match Image In"=w145, "Settings"=w129, "Template Image In"=w128, "select (false=mod))"="select (true= use advanced features\nfase= dont use)", "ROI Descriptor"=w131, "error in (no error)"=w146, "Path In"=w130) -> ("Refnum out"=w125:T9, "Number of Matches"=w126:i32, "Matches"=w127:T13[], "error out"=w124:errorcluster)  [unwired: 5 in]
            n34 = Equal?(x=w126, y=1) -> (x = y?=w181:bool)
            n35 = Array To Cluster(array=w127) -> (cluster=w180:T14)
            n36 = Unbundle By Name(w180) -> ("Matches[0].Correlation Score"=w179:sgl)
            "Current Correlation Score" <- w179
            n37 = Greater?(x=w179, y=w119) -> (0:w178:bool)
            n38 = And(x=w181, y=w178) -> (x .and. y?=w177:bool)
            n39 = case shown="True" w177 {
              tunnel: w125 -> [w673 w706]
              tunnel: w173 -> [_ w708]
              tunnel: w174 -> [_ w707]
              tunnel: w124 -> [_ w705]
              tunnel: w129 -> [_ w704]
              tunnel: [w678 w694] -> w107
              tunnel: [w677 w703] -> w108
              tunnel: [w677 w702] -> w109
              tunnel: [w677 w687] -> w110
              tunnel: [w677 w701] -> w226
              tunnel: [w676 w692] -> w221
              tunnel: [w676 w693] -> w220
              tunnel: [w673 w700] -> w190
              tunnel: [w674 w696] -> w116
              tunnel: w180 -> [_ w699]
              tunnel: w175 -> [_ w698]
              tunnel: w117 -> [_ w697]
              tunnel: [w670 w695] -> w115
              tunnel: w114 -> [_ w691]
              tunnel: w113 -> [_ w690]
              frame False {
                w675 = 0.0
                w676 = sgl 0.0 ("Scale")
                # "Don't Move servo"
                n40 = Bundle(w675, w675) -> (w674:cluster{dbl, dbl})  [unwired: 1 in]
                n41 = Bundle(159.0, 119.0) -> (w670:cluster{dbl, dbl})  [unwired: 1 in]
                n42 = Initialize Array(FALSE, 5 ("dimension size")) -> (w678:bool[])
                n43 = Initialize Array(0.0, 5 ("dimension size")) -> (w677:dbl[])
              }
              frame True {
                n44 = Unbundle By Name(w699) -> ("Matches[0].Position"=w696:cluster{"x":sgl, "y":sgl}, "Matches[0].Bounding Box"=w709:cluster{"x":sgl, "y":sgl}[], "Matches[0].Scale"=w692:sgl, "Matches[0].Score"=w693:sgl)
                n45 = case shown="\"Range 1\", Default" w697 {
                  tunnel: w709 -> [w753 _]
                  tunnel: w708 -> [w749 _]
                  tunnel: w707 -> [w737 _]
                  tunnel: w706 -> [w735 w808]
                  tunnel: w705 -> [w734 _]
                  tunnel: w704 -> [w733 _]
                  tunnel: [w731 w817] -> w686
                  tunnel: [w730 w811] -> w703
                  tunnel: [w729 w812] -> w702
                  tunnel: [w728 w813] -> w687
                  tunnel: [w727 w814] -> w701
                  tunnel: w692 -> [w726 _]
                  tunnel: [w725 w808] -> w700
                  tunnel: w698 -> [w724 _]
                  tunnel: w692 -> [_ w809]
                  tunnel: [w723 w805] -> w695
                  tunnel: w696 -> [w723 _]
                  tunnel: w690 -> [w722 _]
                  frame "Range 1", Default {
                    # "Build ROI for Individual Beacons Based on Main Bounding Box"
                    # "Starting X Lower Bound"
                    # "Beacons to Search For"
                    # "Length of\nIndividual Beacon ROI"
                    # "Length of Bounding Box"
                    # "Draw Bounding Box on Display Image"
                    n46 = Array To Cluster(array=w753) -> (cluster=w754:T15)
                    n47 = Unbundle By Name(w754) -> ("Bounding Box[0].x"=w747:sgl, "Bounding Box[0].y"=w744:sgl, "Bounding Box[2].x"=w750:sgl, "Bounding Box[2].y"=w743:sgl)
                    n48 = Bundle("x"=w747, "y"=w744, "x"=w750, "y"=w743) -> (w752:cluster{"x":sgl, "y":sgl, "x":sgl, "y":sgl})  [unwired: 1 in]
                    n49 = call "IMAQ Overlay Rectangle"("Rectangle"=w752, "Image"=w735) -> ("Image Out"=w732:T9)  [unwired: 8 in, 1 out]
                    n50 = Subtract(x=w750, y=w747) -> (x-y=w751:sgl)
                    n51 = Divide(x=w751, y=w749) -> (x/y=w748:sgl)
                    n52 = Multiply(x=w722, y=w726) -> (x*y=w745:dbl)
                    n53 = Divide(x=w745, y=sgl 100.0) -> (x/y=w740:dbl)
                    n54 = Subtract(x=w744, y=w740) -> (x-y=w742:dbl)
                    n55 = Add(x=w743, y=w740) -> (x+y=w741:dbl)
                    n56 = for {
                      N: 5 -> [_]
                      tunnel: w737 -> [w800] mode=indexing
                      shift-right: [w794] -> _
                      shift-left: w747 -> [w799]
                      tunnel: w748 -> [w798]
                      tunnel: w742 -> [w791]
                      tunnel: w741 -> [w790]
                      tunnel: [w797] -> w736 mode=indexing
                      tunnel: w740 -> [w792]
                      # "Divide Bounding Box"
                      # "Upper Bound of Current is\nLower Bound for Next"
                      n57 = case shown="True" w800 {
                        tunnel: w799 -> [w801 w802]
                        tunnel: w798 -> [_ w804]
                        tunnel: [w801 w803] -> w794
                        tunnel: [w801 w802] -> w796
                        frame False {
                          # "Don't Care"
                        }
                        frame True {
                          # "X Lower Bound"
                          n58 = Add(x=w802, y=w804) -> (x+y=w803:sgl)
                        }
                      }
                      n59 = Subtract(x=w796, y=w792) -> (x-y=w795:dbl)
                      n60 = Add(x=w794, y=w792) -> (x+y=w793:dbl)
                      n61 = call "Bound_RO_R_R0I.vi"("Bottom Right - Y"=w790, "Right - X"=w793, "Top Left - Y"=w791, "Top  Left - x"=w795) -> ("ROI Descriptor"=w797:T12)  [unwired: 7 in]
                    }
                    n62 = for {
                      N: 5 -> [_]
                      tunnel: w735 -> [w767]
                      tunnel: w734 -> [w766]
                      tunnel: w736 -> [w759] mode=indexing
                      tunnel: w724 -> [w765] mode=indexing
                      tunnel: [w764] -> w730 mode=indexing
                      tunnel: [w763] -> w729 mode=indexing
                      tunnel: [w762] -> w731 mode=indexing
                      tunnel: w737 -> [w761] mode=indexing
                      tunnel: w733 -> [w760]
                      shift-right: [w757] -> w725
                      shift-left: w732 -> [w758]
                      tunnel: [w756] -> w728 mode=indexing
                      tunnel: [w755] -> w727 mode=indexing
                      n63 = case shown="True" w761 {
                        tunnel: w767 -> [_ w782]
                        tunnel: w766 -> [_ w781]
                        tunnel: w759 -> [_ w780]
                        tunnel: w765 -> [_ w779]
                        tunnel: [w768 w775] -> w764
                        tunnel: [w768 w774] -> w763
                        tunnel: [FALSE w773] -> w762
                        tunnel: w760 -> [_ w772]
                        tunnel: [w768 w771] -> w756
                        tunnel: [w768 w770] -> w755
                        frame False {
                          w768 = sgl 0.0 ("x")
                        }
                        frame True {
                          n64 = call "Sub Beacon Pattern Match"("Image In"=w782, "ROI Descriptor (Geometric Matching 1)"=w780, "Settings (Geometric Matching 1)"=w772, "Template File Path (Geometric Matching 1)"=w779, "error in"=w781) -> ("Matches (Geometric Matching 1)"=w776:T13[], "Number of Matches (Geometric Matching 1)"=w777:i32)  [unwired: 19 in, 2 out]
                          n65 = Equal?(x=w777, y=1) -> (x = y?=w773:bool)
                          n66 = case shown="True" w773 {
                            tunnel: w776 -> [_ w788]
                            tunnel: [w783 w787] -> w775
                            tunnel: [w783 w786] -> w774
                            tunnel: [w783 w785] -> w771
                            tunnel: [w783 w784] -> w770
                            frame False {
                              w783 = sgl 0.0 ("x")
                            }
                            frame True {
                              n67 = Array To Cluster(array=w788) -> (cluster=w789:T16)
                              n68 = Unbundle By Name(w789) -> ("Matches (Geometric Matching 1)[0].Position.x"=w787:sgl, "Matches (Geometric Matching 1)[0].Position.y"=w786:sgl, "Matches (Geometric Matching 1)[0].Scale"=w785:sgl, "Matches (Geometric Matching 1)[0].Score"=w784:sgl)
                            }
                          }
                        }
                      }
                      n69 = call "IMAQ Overlay ROI"("ROI Descriptor"=w759, "Image"=w758) -> ("Image Out"=w757:T9)  [unwired: 8 in, 1 out]
                    }
                    "Horiztonall Beacon \nCushion (pixels)" <- w722
                  }
                  frame "Range 0" {
                    w810 = sgl 0.0
                    w816 = FALSE
                    # "Don't Move servo"
                    # "Insert Current Scale into index 0"
                    n70 = Bundle(159.0, 119.0) -> (w805:cluster{dbl, dbl})  [unwired: 1 in]
                    n71 = Build Array(TRUE, w816, w816, w816, w816) -> (w817:bool[])
                    n72 = Build Array(w809, w810, w810, w810, w810) -> (w813:sgl[])
                    n73 = Build Array(w810, w810, w810, w810, w810) -> (w812:sgl[])
                    n74 = Build Array(w810, w810, w810, w810, w810) -> (w814:sgl[])
                    n75 = Build Array(w810, w810, w810, w810, w810) -> (w811:sgl[])
                  }
                }
                n76 = Boolean To (0,1)(Boolean=w686) -> (0, 1=w685:i16[])
                n77 = Add Array Elements(numeric array=w685) -> (sum=w684:i16)
                n78 = Add Array Elements(numeric array=w687) -> (sum=w689:sgl)
                n79 = Divide(x=w689, y=w684) -> (x/y=w688:sgl)
                n80 = for {
                  N: 5 -> [_]
                  tunnel: w688 -> [w714]
                  tunnel: w686 -> [w713] mode=indexing
                  tunnel: [w712] -> w694 mode=indexing
                  tunnel: w687 -> [w711] mode=indexing
                  tunnel: w691 -> [w710]
                  # "Check if Scale is within threshold of main,\ndsicard if not"
                  n81 = case shown="True" w713 {
                    selector: w713 -> [w715 _]
                    tunnel: w711 -> [_ w721]
                    tunnel: w714 -> [_ w720]
                    tunnel: [w715 w717] -> w712
                    tunnel: w710 -> [_ w716]
                    frame False {
                    }
                    frame True {
                      n82 = Subtract(x=w721, y=w720) -> (x-y=w719:sgl)
                      n83 = Absolute Value(x=w719) -> (abs(x)=w718:sgl)
                      n84 = Less?(x=w718, y=w716) -> (x < y?=w717:bool)
                    }
                  }
                }
              }
            }
            "Beacons Found" <- w107
            "X Coordinates" <- w108
            "Y Coordinates" <- w109
            "Beacon - Scales" <- w110
            "beacon - Scores" <- w226
            "Current  Scale" <- w221
            "Current  Score" <- w220
            n85 = shared-variable "RT myRIO Target - Overlord\\Localization_Variables_r0.lvlib\\RIGHT_BEACON_Scales"(w110) -> ()  [unwired: 1 in, 1 out]
            n86 = shared-variable "RT myRIO Target - Overlord\\Localization_Variables_r0.lvlib\\RIGHT_BEACON_X_array"(w108) -> ()  [unwired: 1 in, 1 out]
            n87 = shared-variable "RT myRIO Target - Overlord\\Localization_Variables_r0.lvlib\\RIGHT_BEACON_Y_array"(w109) -> ()  [unwired: 1 in, 1 out]
            n88 = shared-variable "RT myRIO Target - Overlord\\Localization_Variables_r0.lvlib\\RIGHT_BEACON_BOOL_array"(w107) -> ()  [unwired: 1 in, 1 out]
            n89 = Boolean To (0,1)(Boolean=w107) -> (0, 1=w228:i16[])
            n90 = Add Array Elements(numeric array=w228) -> (sum=w227:i16)
            n91 = Greater Or Equal?(x=w227, y=w172) -> (x >= y?=w163:bool)
            "Current Valid?" <- w163
            n92 = local read "History Size"() -> (w212:i32)
            n93 = Decrement(x=w212) -> (x-1=w225:i32)
            n94 = for {
              N: w212 -> [_]
              shift-right: [w648] -> w183
              shift-left: w224 -> [w636]
              tunnel: w225 -> [w644]
              shift-right: [w641] -> w151
              shift-left: w223 -> [w643]
              shift-right: [w640] -> w182
              shift-left: w222 -> [w642]
              tunnel: w221 -> [w639]
              tunnel: w220 -> [w638]
              tunnel: w163 -> [w637]
              i -> [w647]
              # "Reverse Index"
              n95 = Subtract(x=w644, y=w647) -> (x-y=w645:i32)
              n96 = Equal To 0?(x=w645) -> (x = 0?=w646:bool)
              n97 = case shown="True" w646 {
                tunnel: w645 -> [w649 w668]
                tunnel: w636 -> [w659 w661]
                tunnel: [w657 w660] -> w648
                tunnel: w637 -> [_ w669]
                tunnel: w643 -> [w654 w667]
                tunnel: w642 -> [w653 w666]
                tunnel: [w652 w664] -> w641
                tunnel: [w651 w665] -> w640
                tunnel: w639 -> [_ w663]
                tunnel: w638 -> [_ w662]
                frame False {
                  # "Shift Old"
                  n98 = Decrement(x=w649) -> (x-1=w650:i32)
                  n99 = Index Array(array=w659, index=w650) -> (element=w658:bool)
                  n100 = Index Array(array=w654, index=w650) -> (element=w656:dbl)
                  n101 = Index Array(array=w653, index=w650) -> (element=w655:dbl)
                  n102 = Replace Array Subset(array=w659, new element=w658, index=w649) -> (w657:bool[])
                  n103 = Replace Array Subset(array=w654, new element=w656, index=w649) -> (w652:dbl[])
                  n104 = Replace Array Subset(array=w653, new element=w655, index=w649) -> (w651:dbl[])
                }
                frame True {
                  # "Score"
                  # "Scale"
                  # "Valid"
                  # "insert New"
                  n105 = Replace Array Subset(array=w667, new element=w663, index=w668) -> (w664:dbl[])
                  n106 = Replace Array Subset(array=w666, new element=w662, index=w668) -> (w665:dbl[])
                  n107 = Replace Array Subset(array=w661, new element=w669, index=w668) -> (w660:bool[])
                }
              }
            }
            n108 = Boolean To (0,1)(Boolean=w183) -> (0, 1=w218:i16[])
            n109 = Add Array Elements(numeric array=w218) -> (sum=w217:i16)
            n110 = Greater Or Equal?(x=w217, y="Valid Treshold\nfor Lock") -> (x >= y?=w111:bool)
            "Lock Status" <- w111
            n111 = shared-variable "RT myRIO Target - Overlord\\Localization_Variables_r0.lvlib\\Image Lock - R"(w111) -> ()  [unwired: 1 in, 1 out]
            n112 = Initialize Array(u8 0, "Max Window\n for Avg") -> (w215:u8[])
            n113 = while {
              shift-right: [w619] -> w211
              shift-left: w215 -> [w621]
              tunnel: w183 -> [w627] mode=indexing
              shift-right: [w625] -> w208
              shift-left: u8 0 -> [w628]
              tunnel: w212 -> [w626]
              tunnel: "Max Window\n for Avg" -> [w618]
              i -> [w620]
              stop <- w622 stop-if-true
              # "Grab Last 'X' Valid Indexes"
              n114 = case shown="True" w627 {
                tunnel: w628 -> [w630 w632]
                tunnel: [w630 w635] -> w625
                tunnel: w621 -> [w629 w634]
                tunnel: w620 -> [_ w633]
                tunnel: [w629 w631] -> w619
                frame False {
                }
                frame True {
                  # "Update Index\nto use"
                  # "Increment\nValid Count"
                  n115 = Replace Array Subset(array=w634, new element=w633, index=w632) -> (w631:u8[])
                  n116 = Increment(x=w632) -> (x+1=w635:u8)
                }
              }
              n117 = Greater?(x=w620, y=w626) -> (0:w623:bool)
              n118 = Greater Or Equal?(x=w625, y=w618) -> (x >= y?=w624:bool)
              n119 = Or(x=w624, y=w623) -> (x .or. y?=w622:bool)
            }
            n120 = Greater Or Equal?(x=w208, y=u8 2) -> (x >= y?=w209:bool)
            n121 = case shown="True" w209 {
              tunnel: w208 -> [_ w602]
              tunnel: w211 -> [_ w608]
              tunnel: w151 -> [_ w607]
              tunnel: w182 -> [_ w606]
              tunnel: ["Avg Scale - Last" w600] -> w171
              tunnel: ["Avg Score - Last" w599] -> w170
              frame False {
              }
              frame True {
                w605 = 0.0
                n122 = for {
                  N: w602 -> [_]
                  tunnel: w608 -> [w615] mode=indexing
                  tunnel: w607 -> [w617]
                  tunnel: w606 -> [w616]
                  shift-right: [w613] -> w604
                  shift-left: w605 -> [w611]
                  shift-right: [w614] -> w603
                  shift-left: w605 -> [w610]
                  # "Fetch Last Valid Values"
                  n123 = Index Array(array=w617, index=w615) -> (element=w612:dbl)
                  n124 = Index Array(array=w616, index=w615) -> (element=w609:dbl)
                  n125 = Add(x=w612, y=w611) -> (x+y=w613:dbl)
                  n126 = Add(x=w609, y=w610) -> (x+y=w614:dbl)
                }
                n127 = To Double Precision Float(number=w602) -> (double precision float=w601:dbl)
                n128 = Divide(x=w604, y=w601) -> (x/y=w600:dbl)
                n129 = Divide(x=w603, y=w601) -> (x/y=w599:dbl)
                n130 = local write "Avg Scale - Last"(w600) -> ()
                n131 = local write "Avg Score - Last"(w599) -> ()
              }
            }
            "Avg Score" <- w170
            "Avg Scale" <- w171
            n132 = And(x=w111, y=w149) -> (x .and. y?=w150:bool)
            n133 = case shown="False" w150 {
              selector: w150 -> [_ w232]
              tunnel: [w230 w231] -> w148
              tunnel: w149 -> [w230 _]
              frame False {
              }
              frame True {
                # "Pull Down Start Up \nFlag"
                n134 = Not(x=w232) -> (.not. x?=w231:bool)
              }
            }
            n135 = Unbundle By Name(w129) -> ("Minimum Match Score"=w168:sgl, "Range Settings"=w195:T7[], "Curve Parameters"=w165:T6)
            n136 = Index Array(array=w195, index=u32 1) -> (element=w196:T7)
            n137 = Unbundle(w196) -> ("Min"=w167:dbl, "Max"=w166:dbl)  [unwired: 1 out]
            n138 = case shown="False" w148 {
              tunnel: w111 -> [w255 _]
              tunnel: w117 -> [w254 w559]
              tunnel: w171 -> [w253 _]
              tunnel: [w237 w559] -> w153
              tunnel: w171 -> [w252 _]
              tunnel: w170 -> [w251 _]
              tunnel: "Score\nCushion" -> [w250 _]
              tunnel: w168 -> [w249 w556]
              tunnel: w167 -> [w248 w555]
              tunnel: w166 -> [w247 w554]
              tunnel: w116 -> [w246 _]
              tunnel: w131 -> [w245 w558]
              tunnel: w165 -> [w244 _]
              tunnel: w165 -> [w243 w557]
              tunnel: [w242 w556] -> w157
              tunnel: [w241 w555] -> w155
              tunnel: [w240 w554] -> w156
              tunnel: [w239 w558] -> w154
              tunnel: [w238 w557] -> w162
              tunnel: [w236 FALSE] -> w164
              tunnel: w163 -> [w235 _]
              tunnel: w151 -> [w234 w552]
              tunnel: [w233 w552] -> w152
              frame False {
                # "Current Template"
                # "Image Lock?"
                n139 = case shown="False" w255 {
                  tunnel: w254 -> [_ w347]
                  tunnel: [w257 w310] -> w237
                  tunnel: w253 -> [_ w348]
                  tunnel: w252 -> [_ w346]
                  tunnel: w251 -> [_ w344]
                  tunnel: w250 -> [_ w343]
                  tunnel: w249 -> [_ w342]
                  tunnel: w248 -> [_ w341]
                  tunnel: w247 -> [_ w340]
                  tunnel: w246 -> [_ w339]
                  tunnel: w245 -> [_ w338]
                  tunnel: w244 -> [_ w335]
                  tunnel: w243 -> [w262 w320]
                  tunnel: [w261 w315] -> w238
                  tunnel: [w273 w314] -> w239
                  tunnel: [w282 w313] -> w242
                  tunnel: [w281 w312] -> w241
                  tunnel: [w280 w311] -> w240
                  tunnel: [FALSE w309] -> w236
                  tunnel: w235 -> [_ w308]
                  tunnel: w234 -> [w259 w307]
                  tunnel: [w259 w306] -> w233
                  frame False {
                    # "Apply default settings for the selected template"
                    # "Initial ROI Descriptor"
                    # "Check Other Camera?"
                    n140 = shared-variable "RT myRIO Target - Overlord\\Localization_Variables_r0.lvlib\\Image Lock - L"() -> (w256:bool)  [unwired: 1 in, 1 out]
                    n141 = case shown="True" w256 {
                      tunnel: [w288 w305] -> w257
                      frame False {
                        # "No Lock Available, Choose Based off last position"
                        n142 = shared-variable "RT myRIO Target - Overlord\\Localization_Variables_r0.lvlib\\Last Robot Position"() -> (w287:cluster{"X":sgl, "Y":sgl})  [unwired: 1 in, 1 out]
                        n143 = Unbundle By Name(w287) -> ("X"=w289:sgl)
                        n144 = Less?(x=w289, y=sgl 3.0) -> (x < y?=w290:bool)
                        n145 = case shown="False" w290 {
                          tunnel: [w293 T4."Range 0" ("Current Template")] -> w288
                          tunnel: w289 -> [w292 _]
                          frame False {
                            n146 = Less?(x=w292, y=sgl 5.0) -> (x < y?=w294:bool)
                            n147 = case shown="True" w294 {
                              tunnel: [w297 T4."Range 1" ("Current Template")] -> w293
                              tunnel: w292 -> [w299 _]
                              frame False {
                                n148 = Less?(x=w299, y=sgl 10.0) -> (x < y?=w296:bool)
                                n149 = case shown="False" w296 {
                                tunnel: [T4."Range 3" ("Current Template") T4."Range 2" ("Current Template")] -> w297
                                frame False {
                                }
                                frame True {
                                }
                                }
                              }
                              frame True {
                              }
                            }
                          }
                          frame True {
                          }
                        }
                      }
                      frame True {
                        # "If other Camera is Locked, Use its template and apply default settings for that template"
                        n150 = shared-variable "RT myRIO Target - Overlord\\Localization_Variables_r0.lvlib\\Info - Left"() -> (w304:T5)  [unwired: 1 in, 1 out]
                        n151 = Unbundle By Name(w304) -> ("Current Template"=w305:T4)
                      }
                    }
                    n152 = case shown="\"Range 2\"" w257 {
                      tunnel: [w283 w284 w285 w286] -> w258
                      frame "Range 1", Default {
                        n153 = local read "Range 1 Default\nSetting Values"() -> (w283:T1)
                      }
                      frame "Range 2" {
                        n154 = local read "Range 2 Default\nSetting Values"() -> (w284:T1)
                      }
                      frame "Range 3" {
                        n155 = local read "Range 3 Default\nSetting Values"() -> (w285:T1)
                      }
                      frame "Range 0" {
                        n156 = local read "Range 0 Default\nSetting Values"() -> (w286:T1)
                      }
                    }
                    n157 = Unbundle By Name(w258) -> ("Min Score"=w282:dbl, "Min Scale"=w281:dbl, "Max Scale"=w280:dbl, "Curve Parameters"=w263:T17)
                    n158 = Bundle(0, 0, 640, 480, 0) -> (w279:cluster{i32, i32, i32, i32, i32})  [unwired: 1 in]
                    n159 = call "IMAQ Convert Rectangle to ROI"("Rectangle"=w279) -> ("ROI Descriptor"=w273:T12)  [unwired: 8 in, 1 out]
                    n160 = Unbundle By Name(w263) -> ("Min Length"=w267:i32, "Row Search Step"=w268:i32, "Col Search Step"=w269:i32)
                    n161 = Unbundle(w262) -> ("Extraction Mode"=w264:u32, "Edge Threshold"=w265:i32, "Edge Filter Size"=w266:u32, "Max Endpoint Gap"=w270:i32, "Closed"=w271:bool, "Subpixel"=w272:bool)  [unwired: 3 out]
                    n162 = Bundle("Extraction Mode"=w264, "Edge Threshold"=w265, "Edge Filter Size"=w266, "Min Length"=w267, "Row Search Step"=w268, "Col Search Step"=w269, "Max Endpoint Gap"=w270, "Closed"=w271, "Subpixel"=w272) -> (w261:T18)  [unwired: 1 in]
                  }
                  frame True {
                    # "Update Search Settings"
                    # "Next State"
                    # "Changing Templates?"
                    # "Update Template"
                    n163 = case shown="\"Range 1\", Default" w347 {
                      selector: w347 -> [w484 w515 w533 w548]
                      tunnel: w348 -> [w485 w517 w534 w549]
                      tunnel: [w486 w516 w532 w547] -> w310
                      tunnel: [w500 w506 w526 w541] -> w345
                      tunnel: [w499 w505 w525 w540] -> w337
                      tunnel: [w498 w504 w524 w539] -> w336
                      tunnel: [w497 w507 w530 w545] -> w331
                      tunnel: [w496 w509 w527 w542] -> w323
                      tunnel: [w495 w510 w528 w543] -> w322
                      tunnel: [w494 w513 w529 w544] -> w321
                      frame "Range 1", Default {
                        # "Next Template"
                        # "Next Template"
                        n164 = local read "Range 1 Default\nSetting Values"() -> (w501:T1)
                        n165 = Unbundle By Name(w501) -> ("Lower Transition Scale"=w482:sgl, "Upper Transition Scale"=w483:sgl, "ROI Vertical"=w498:dbl, "ROI Horizontal"=w499:dbl, "Scale Cushion"=w500:dbl, "Curve Parameters"=w497:T17, "Min Score"=w496:dbl, "Min Scale"=w495:dbl, "Max Scale"=w494:dbl)
                        n166 = Less?(x=w485, y=w482) -> (x < y?=w493:bool)
                        n167 = Not(x=w493) -> (.not. x?=w492:bool)
                        n168 = Select(t=w484, s=w492, f=T4."Range 2" ("Initial Template 2")) -> (s? t:f=w489:T4)
                        n169 = Greater?(x=w485, y=w483) -> (0:w491:bool)
                        n170 = Not(x=w491) -> (.not. x?=w490:bool)
                        n171 = Select(t=w489, s=w490, f=T4."Range 0" ("Initial Template 2")) -> (s? t:f=w486:T4)
                      }
                      frame "Range 2" {
                        # "Next Template"
                        # "Next Template"
                        n172 = local read "Range 2 Default\nSetting Values"() -> (w514:T1)
                        n173 = Unbundle By Name(w514) -> ("Lower Transition Scale"=w512:sgl, "Upper Transition Scale"=w511:sgl, "ROI Vertical"=w504:dbl, "ROI Horizontal"=w505:dbl, "Scale Cushion"=w506:dbl, "Curve Parameters"=w507:T17, "Min Score"=w509:dbl, "Min Scale"=w510:dbl, "Max Scale"=w513:dbl)
                        n174 = Less?(x=w517, y=w512) -> (x < y?=w521:bool)
                        n175 = Not(x=w521) -> (.not. x?=w520:bool)
                        n176 = Select(t=w515, s=w520, f=T4."Range 3" ("Initial Template 2")) -> (s? t:f=w508:T4)
                        n177 = Greater?(x=w517, y=w511) -> (0:w519:bool)
                        n178 = Not(x=w519) -> (.not. x?=w518:bool)
                        n179 = Select(t=w508, s=w518, f=T4."Range 1" ("Initial Template 2")) -> (s? t:f=w516:T4)
                      }
                      frame "Range 3" {
                        # "Next Template"
                        n180 = local read "Range 3 Default\nSetting Values"() -> (w531:T1)
                        n181 = Unbundle By Name(w531) -> ("Upper Transition Scale"=w523:sgl, "ROI Vertical"=w524:dbl, "ROI Horizontal"=w525:dbl, "Scale Cushion"=w526:dbl, "Curve Parameters"=w530:T17, "Min Score"=w527:dbl, "Min Scale"=w528:dbl, "Max Scale"=w529:dbl)  [unwired: 1 out]
                        n182 = Greater?(x=w534, y=w523) -> (0:w536:bool)
                        n183 = Not(x=w536) -> (.not. x?=w535:bool)
                        n184 = Select(t=w533, s=w535, f=T4."Range 2" ("Initial Template 2")) -> (s? t:f=w532:T4)
                      }
                      frame "Range 0" {
                        # "Next Template"
                        n185 = local read "Range 0 Default\nSetting Values"() -> (w546:T1)
                        n186 = Unbundle By Name(w546) -> ("Lower Transition Scale"=w537:sgl, "ROI Vertical"=w539:dbl, "ROI Horizontal"=w540:dbl, "Scale Cushion"=w541:dbl, "Curve Parameters"=w545:T17, "Min Score"=w542:dbl, "Min Scale"=w543:dbl, "Max Scale"=w544:dbl)  [unwired: 1 out]
                        n187 = Less?(x=w549, y=w537) -> (x < y?=w551:bool)
                        n188 = Not(x=w551) -> (.not. x?=w550:bool)
                        n189 = Select(t=w548, s=w550, f=T4."Range 1" ("Initial Template 2")) -> (s? t:f=w547:T4)
                      }
                    }
                    n190 = Unbundle By Name(w331) -> ("Min Length"=w330:i32, "Row Search Step"=w329:i32, "Col Search Step"=w328:i32)
                    n191 = Unbundle(w335) -> ("Extraction Mode"=w334:u32, "Edge Threshold"=w333:i32, "Edge Filter Size"=w332:u32, "Max Endpoint Gap"=w327:i32, "Closed"=w326:bool, "Subpixel"=w325:bool)  [unwired: 3 out]
                    n192 = Bundle("Extraction Mode"=w334, "Edge Threshold"=w333, "Edge Filter Size"=w332, "Min Length"=w330, "Row Search Step"=w329, "Col Search Step"=w328, "Max Endpoint Gap"=w327, "Closed"=w326, "Subpixel"=w325) -> (w324:T18)  [unwired: 1 in]
                    n193 = Not Equal?(x=w310, y=w347) -> (x != y?=w309:bool)
                    n194 = case shown="True" w309 {
                      tunnel: w308 -> [w371 _]
                      tunnel: w346 -> [w370 _]
                      tunnel: w345 -> [w369 _]
                      tunnel: w344 -> [w368 _]
                      tunnel: w343 -> [w367 _]
                      tunnel: w342 -> [w366 _]
                      tunnel: w341 -> [w365 _]
                      tunnel: w340 -> [w364 _]
                      tunnel: w339 -> [w363 _]
                      tunnel: w338 -> [w362 _]
                      tunnel: w337 -> [w361 _]
                      tunnel: w336 -> [w360 _]
                      tunnel: [w358 w445] -> w313
                      tunnel: w324 -> [w349 _]
                      tunnel: [w357 w444] -> w312
                      tunnel: [w356 w443] -> w311
                      tunnel: w323 -> [_ _]
                      tunnel: w322 -> [_ _]
                      tunnel: w321 -> [_ _]
                      tunnel: w310 -> [_ w447]
                      tunnel: w320 -> [_ w460]
                      tunnel: [w350 w459] -> w315
                      tunnel: [w355 w454] -> w319
                      tunnel: [w354 w453] -> w318
                      tunnel: [w353 w437] -> w317
                      tunnel: [w352 w438] -> w316
                      tunnel: w307 -> [w351 w440]
                      tunnel: [w351 w439] -> w306
                      frame False {
                        w359 = 500.0 ("y")
                        # "Current Valid?"
                        # "********"
                        # "Apply Limit to Score"
                        # "Score out"
                        # "Apply Limits to ROI"
                        n195 = case shown="False" w371 {
                          tunnel: w368 -> [_ w420]
                          tunnel: w367 -> [_ w419]
                          tunnel: w370 -> [_ w410]
                          tunnel: w369 -> [w399 w418]
                          tunnel: [w382 w413] -> w355
                          tunnel: [w381 w409] -> w354
                          tunnel: [w380 w412] -> w353
                          tunnel: [w379 w411] -> w352
                          tunnel: [w395 w408] -> w372
                          tunnel: [w394 w407] -> w357
                          tunnel: [w393 w406] -> w356
                          tunnel: w362 -> [w391 _]
                          tunnel: w366 -> [w378 _]
                          tunnel: w365 -> [w377 _]
                          tunnel: w364 -> [w376 _]
                          tunnel: w363 -> [_ w405]
                          tunnel: w361 -> [_ w401]
                          tunnel: w360 -> [_ w402]
                          tunnel: [w374 w400] -> w350
                          tunnel: w349 -> [w374 w400]
                          frame False {
                            # "Current Match was Invalid"
                            n196 = Divide(x=w399, y=sgl 3.0) -> (x/y=w397:dbl)
                            n197 = Subtract(x=w377, y=w397) -> (x-y=w394:dbl)
                            n198 = Add(x=w376, y=w397) -> (x+y=w393:dbl)
                            n199 = Subtract(x=w378, y="Score Decay \nFactor 2") -> (x-y=w395:dbl)
                            n200 = call "IMAQ Convert ROI to Rectangle"("ROI Descriptor"=w391) -> ("Rectangle"=w392:T19)  [unwired: 8 in, 1 out]
                            n201 = Unbundle By Name(w392) -> ("Left"=w386:i32, "Top"=w385:i32, "Right"=w384:i32, "Bottom"=w383:i32)
                            n202 = To Long Integer(number="ROI Decay Factor (px)") -> (32bit integer=w388:i32)
                            n203 = Divide(x="ROI Decay Factor (px)", y=sgl 10.0) -> (x/y=w390:dbl)
                            n204 = Subtract(x=w386, y=w388) -> (x-y=w382:i32)
                            n205 = Add(x=w384, y=w388) -> (x+y=w380:i32)
                            n206 = To Long Integer(number=w390) -> (32bit integer=w387:i32)
                            n207 = Subtract(x=w385, y=w387) -> (x-y=w381:i32)
                            n208 = Add(x=w383, y=w387) -> (x+y=w379:i32)
                          }
                          frame True {
                            (unwired) sgl 109.0 ("x")
                            (unwired) sgl 159.0 ("x")
                            # "Current Match was Valid"
                            # "Center of Image"
                            # "Main ROI"
                            # "Horizontal Scale \n(smaller number = smaller ROI)"
                            n209 = Subtract(x=w420, y=w419) -> (x-y=w408:dbl)
                            n210 = case shown="0, Default" "ROBOT STATE\n(fwd, bwd, neither) 2" {
                              tunnel: w410 -> [w425 w430 w435]
                              tunnel: [w424 w426 w431] -> w406
                              tunnel: w418 -> [w422 w429 w434]
                              tunnel: [w423 w427 w432] -> w407
                              frame 0, Default {
                                n211 = Subtract(x=w425, y=w422) -> (x-y=w423:dbl)
                                n212 = Add(x=w422, y=w425) -> (x+y=w424:dbl)
                              }
                              frame 1 {
                                n213 = Subtract(x=w430, y=5.0) -> (x-y=w427:dbl)
                                n214 = Add(x=w429, y=w430) -> (x+y=w426:dbl)
                              }
                              frame -1 {
                                n215 = Subtract(x=w435, y=w434) -> (x-y=w432:dbl)
                                n216 = Add(x=5.0 ("y"), y=w435) -> (x+y=w431:dbl)
                              }
                            }
                            n217 = Unbundle(w405) -> ("x"=w404:dbl, "y"=w403:dbl)
                            n218 = Divide(x=w410, y=w402) -> (x/y=w416:dbl)
                            n219 = Multiply(x=w410, y=w401) -> (x*y=w414:dbl)
                            n220 = Divide(x=w414, y=sgl 2.0) -> (x/y=w417:dbl)
                            n221 = Add(x=w403, y=w416) -> (x+y=w411:dbl)
                            n222 = Subtract(x=w403, y=w416) -> (x-y=w409:dbl)
                            n223 = Subtract(x=w404, y=w417) -> (x-y=w413:dbl)
                            n224 = Add(x=w417, y=w404) -> (x+y=w412:dbl)
                          }
                        }
                        n225 = Greater?(x=w372, y=w359) -> (0:w373:bool)
                        n226 = Select(t=w372, s=w373, f=w359) -> (s? t:f=w358:dbl)
                      }
                      frame True {
                        w450 = sgl 125.0 ("x")
                        w451 = sgl 109.0 ("x")
                        w452 = sgl 159.0 ("x")
                        # "Reset Scale to 100"
                        # "\"Start Scale\""
                        # "Center of Image"
                        # "Main ROI"
                        # "Horizontal Scale \n(smaller number = smaller ROI)"
                        # "Apply New Curve Parameters"
                        # "Next State"
                        # "Changing States - Apply Initial Settings for that State"
                        n227 = local read "History Size"() -> (w441:i32)
                        n228 = case shown="\"Range 3\"" w447 {
                          tunnel: [w475 w477 w479 w481] -> w446
                          tunnel: [50.0 ("Avg Scale - Last") 90.0 ("Avg Scale - Last") 90.0 ("Avg Scale - Last") 90.0 ("Avg Scale - Last")] -> w436
                          frame "Range 1", Default {
                            n229 = local read "Range 1 Default\nSetting Values"() -> (w475:T1)
                          }
                          frame "Range 2" {
                            n230 = local read "Range 2 Default\nSetting Values"() -> (w477:T1)
                          }
                          frame "Range 3" {
                            n231 = local read "Range 3 Default\nSetting Values"() -> (w479:T1)
                          }
                          frame "Range 0" {
                            n232 = local read "Range 0 Default\nSetting Values"() -> (w481:T1)
                          }
                        }
                        n233 = local write "Avg Scale - Last"(w436) -> ()
                        n234 = for {
                          N: w441 -> [_]
                          tunnel: w436 -> [w471]
                          shift-right: [w470] -> w439
                          shift-left: w440 -> [w473]
                          i -> [w472]
                          n235 = Replace Array Subset(array=w473, new element=w471, index=w472) -> (w470:dbl[])
                        }
                        n236 = Unbundle By Name(w446) -> ("Min Score"=w445:dbl, "Min Scale"=w444:dbl, "Max Scale"=w443:dbl, "Curve Parameters"=w442:T17, "ROI Vertical"=w449:dbl, "ROI Horizontal"=w448:dbl)
                        n237 = Unbundle By Name(w442) -> ("Min Length"=w464:i32, "Row Search Step"=w465:i32, "Col Search Step"=w466:i32)
                        n238 = Unbundle(w460) -> ("Extraction Mode"=w461:u32, "Edge Threshold"=w462:i32, "Edge Filter Size"=w463:u32, "Max Endpoint Gap"=w467:i32, "Closed"=w468:bool, "Subpixel"=w469:bool)  [unwired: 3 out]
                        n239 = Bundle("Extraction Mode"=w461, "Edge Threshold"=w462, "Edge Filter Size"=w463, "Min Length"=w464, "Row Search Step"=w465, "Col Search Step"=w466, "Max Endpoint Gap"=w467, "Closed"=w468, "Subpixel"=w469) -> (w459:T18)  [unwired: 1 in]
                        n240 = Divide(x=w450, y=w449) -> (x/y=w457:dbl)
                        n241 = Multiply(x=w450, y=w448) -> (x*y=w455:dbl)
                        n242 = Divide(x=w455, y=sgl 2.0) -> (x/y=w458:dbl)
                        n243 = Add(x=w451, y=w457) -> (x+y=w438:dbl)
                        n244 = Subtract(x=w451, y=w457) -> (x-y=w453:dbl)
                        n245 = Subtract(x=w452, y=w458) -> (x-y=w454:dbl)
                        n246 = Add(x=w458, y=w452) -> (x+y=w437:dbl)
                      }
                    }
                    n247 = call "Bound_RO_R_R0I.vi"("Bottom Right - Y"=w316, "Right - X"=w317, "Top Left - Y"=w318, "Top  Left - x"=w319) -> ("ROI Descriptor"=w314:T12)  [unwired: 7 in]
                  }
                }
              }
              frame True {
              }
            }
            "Next Template" <- w153
            n248 = Less?(x=w157, y="Absolute\nMinimum Score") -> (x < y?=w201:bool)
            n249 = Less?(x=w155, y="Absolute\nMinimum Scale") -> (x < y?=w204:bool)
            n250 = Greater?(x=w156, y="Absolute\nMaximum Scale") -> (0:w207:bool)
            n251 = Greater?(x=w155, y=w156) -> (0:w203:bool)
            n252 = Less?(x=w156, y=w155) -> (x < y?=w206:bool)
            n253 = Select(t="Absolute\nMinimum Score", s=w201, f=w157) -> (s? t:f=w189:dbl)
            "New Min Score" <- w189
            n254 = Or(x=w204, y=w203) -> (x .or. y?=w202:bool)
            n255 = Or(x=w207, y=w206) -> (x .or. y?=w205:bool)
            n256 = Select(t="Absolute\nMinimum Scale", s=w202, f=w155) -> (s? t:f=w188:dbl)
            "New Low Scale" <- w188
            n257 = Select(t="Absolute\nMaximum Scale", s=w205, f=w156) -> (s? t:f=w187:dbl)
            "New high Scale" <- w187
            n258 = Bundle("index"=w194, "Min"=w188, "Max"=w187) -> (w193:cluster{"index":u32, "Min":dbl, "Max":dbl})  [unwired: 1 in]
            n259 = Replace Array Subset(array=w195, new element=w193, index=w194) -> (w192:T7[])
            n260 = Bundle By Name(cluster=w129, "Minimum Match Score"=w189, "Range Settings"=w192, "Curve Parameters"=w162) -> (w191:T8)
            n261 = call "IMAQ Overlay ROI"("ROI Descriptor"=w154, "Image"=w190) -> ("Image Out"=→"Right Image out":T9)  [unwired: 8 in, 1 out]
            n262 = Unbundle By Name(w162) -> ("Min Length"=w161:i32, "Row Search Step Size"=w160:i32, "Col Search Step Size"=w159:i32)
            n263 = Bundle("Min Length"=w161, "Row Search Step Size"=w160, "Col Search Step Size"=w159) -> (w158:T20)  [unwired: 1 in]
            n264 = Bundle("Min Score"=w189, "Min"=w188, "Max"=w187, w158) -> (w186:T21)  [unwired: 1 in]
            n265 = case shown="True" w164 {
              tunnel: w115 -> [w820 w826]
              tunnel: w163 -> [w821 w832]
              tunnel: w107 -> [_ _]
              tunnel: w186 -> [w823 w830]
              tunnel: w111 -> [w822 w833]
              tunnel: w153 -> [w819 w831]
              tunnel: [w818 w829] -> w112
              frame False {
                n266 = Bundle(w822, w821, "Initial Template"=w819, "Position"=w820, w823) -> (w818:T22)  [unwired: 1 in]
              }
              frame True {
                # "Check if Tracking is Available for the Next Template State"
                n267 = local read "Current Template"() -> (w824:T4)
                n268 = Unbundle(w826) -> ("x"=w828:dbl, "y"=w827:dbl)
                n269 = case shown="\"Range 2\"" w831 {
                  tunnel: w828 -> [w838 w847 _ _]
                  tunnel: w827 -> [w834 w846 _ _]
                  tunnel: w826 -> [_ w844 w855 _]
                  tunnel: [w837 w845 w855 w858] -> w825
                  tunnel: w824 -> [w835 w843 _ _]
                  frame "Range 1" {
                    n270 = case shown="\"Range 2\"" w835 {
                      tunnel: w838 -> [w839 w842]
                      tunnel: [w839 w840] -> w836
                      frame "Range 0", Default {
                      }
                      frame "Range 2" {
                        n271 = Add(x=w842, y=-70.0) -> (x+y=w840:dbl)
                      }
                    }
                    n272 = Bundle("x"=w836, "y"=w834) -> (w837:cluster{"x":dbl, "y":dbl})  [unwired: 1 in]
                  }
                  frame "Range 2" {
                    # "Depends on Current State"
                    n273 = case shown="\"Range 3\"" w843 {
                      tunnel: w847 -> [w852 _ _]
                      tunnel: w846 -> [w849 _ _]
                      tunnel: [w848 w853 w854] -> w845
                      tunnel: w844 -> [_ w853 w854]
                      frame "Range 1" {
                        n274 = Add(x=w852, y=70.0) -> (x+y=w850:dbl)
                        n275 = Bundle(w850, "y"=w849) -> (w848:cluster{dbl, "y":dbl})  [unwired: 1 in]
                      }
                      frame "Range 2", Default {
                      }
                      frame "Range 3" {
                      }
                    }
                  }
                  frame "Range 3", Default {
                  }
                  frame "Range 0" {
                    # "Don't Move servo"
                    n276 = Bundle(159.0, 119.0) -> (w858:cluster{dbl, dbl})  [unwired: 1 in]
                  }
                }
                n277 = Bundle(w833, w832, "Initial Template"=w831, "Position"=w825, w830) -> (w829:T22)  [unwired: 1 in]
              }
            }
            "Tracking Info" <- w112
            n278 = shared-variable "RT myRIO Target - Overlord\\Localization_Variables_r0.lvlib\\Info - Right"(w112) -> ()  [unwired: 1 in, 1 out]
          }
          frame #2 {
            n279 = shared-variable "RT myRIO Target - Overlord\\Localization_Variables_r0.lvlib\\Right Servo Angle_Image"(w860) -> ()  [unwired: 1 in, 1 out]
            n280 = shared-variable "RT myRIO Target - Overlord\\Localization_Variables_r0.lvlib\\RIGHT_FLAG"(TRUE ("RIGHT_FLAG")) -> ()  [unwired: 1 in, 1 out]
          }
        }
        "Startup Flag" <- w75
        "Valid Scale History" <- w82
        "Valid Beacon History - in" <- w84
        "Valid Score History" <- w81
        "Current Search Settings" <- w92
        "Current Template" <- w79
      }
    }
    frame #2 {
      n281 = call <vilib>:"IMAQdx Close Camera.vi"("Session In"=w863) -> ()  [unwired: 10 in, 1 out]
    }
  }
